vi "torres hanoi.vi"() -> ()   [LabVIEW 2020]
uses:
  <vilib>/Utility/miscctls.llb/LVPoint32TypeDef.ctl
  <vilib>/Utility/miscctls.llb/LVPositionTypeDef.ctl
  <vilib>/Utility/miscctls.llb/LVBoundsTypeDef.ctl
panel:
  out "?":string
  out "solucion de inicio a final 5":string
  out "solucion de inicio a final 4":string
  in  "?":bool
  out "solucion de inicio a final 3":string
  out "result":bool
  out "Position 1":T1
  out "# de movimientos":dbl
  out "Position 2":T1
  out "Position 3":T1
  out "Position 4":T1
  out "Position 5":T1
  out "Position":T1
  in  "seleccione  # de discos:":u16(ring) items=["3"=3, "4"=4, "5"=5]
  out "Coords":T2
  in  "?":bool
  out "disco5":bool
  out "disco4":bool
  out "disco3":bool
  out "disco2":bool
  out "disco1":bool
  out "final":bool
  out "medio":bool
  out "inicio":bool
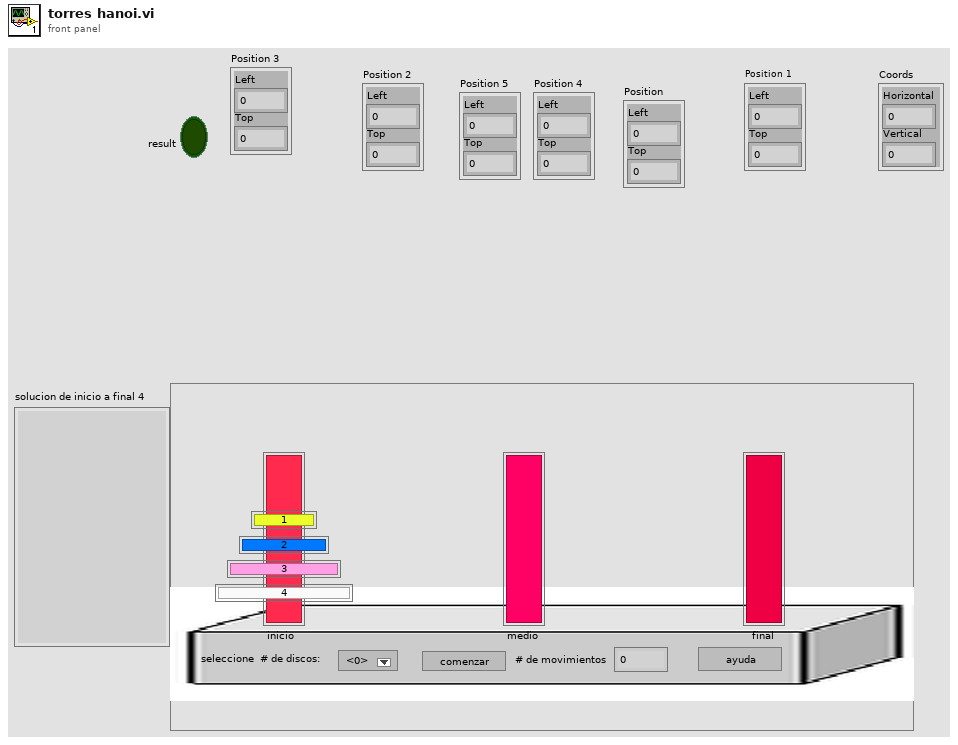
[diagram p1: front panel]
types:
  T1 = typedef "LVPositionTypeDef.ctl" = cluster{"Left":i32, "Top":i32}
  T2 = typedef "LVPoint32TypeDef.ctl" = cluster{"Horizontal":i32, "Vertical":i32}
  T3 = typedef "LVBoundsTypeDef.ctl" = cluster{"Width":u32, "Height":u32}
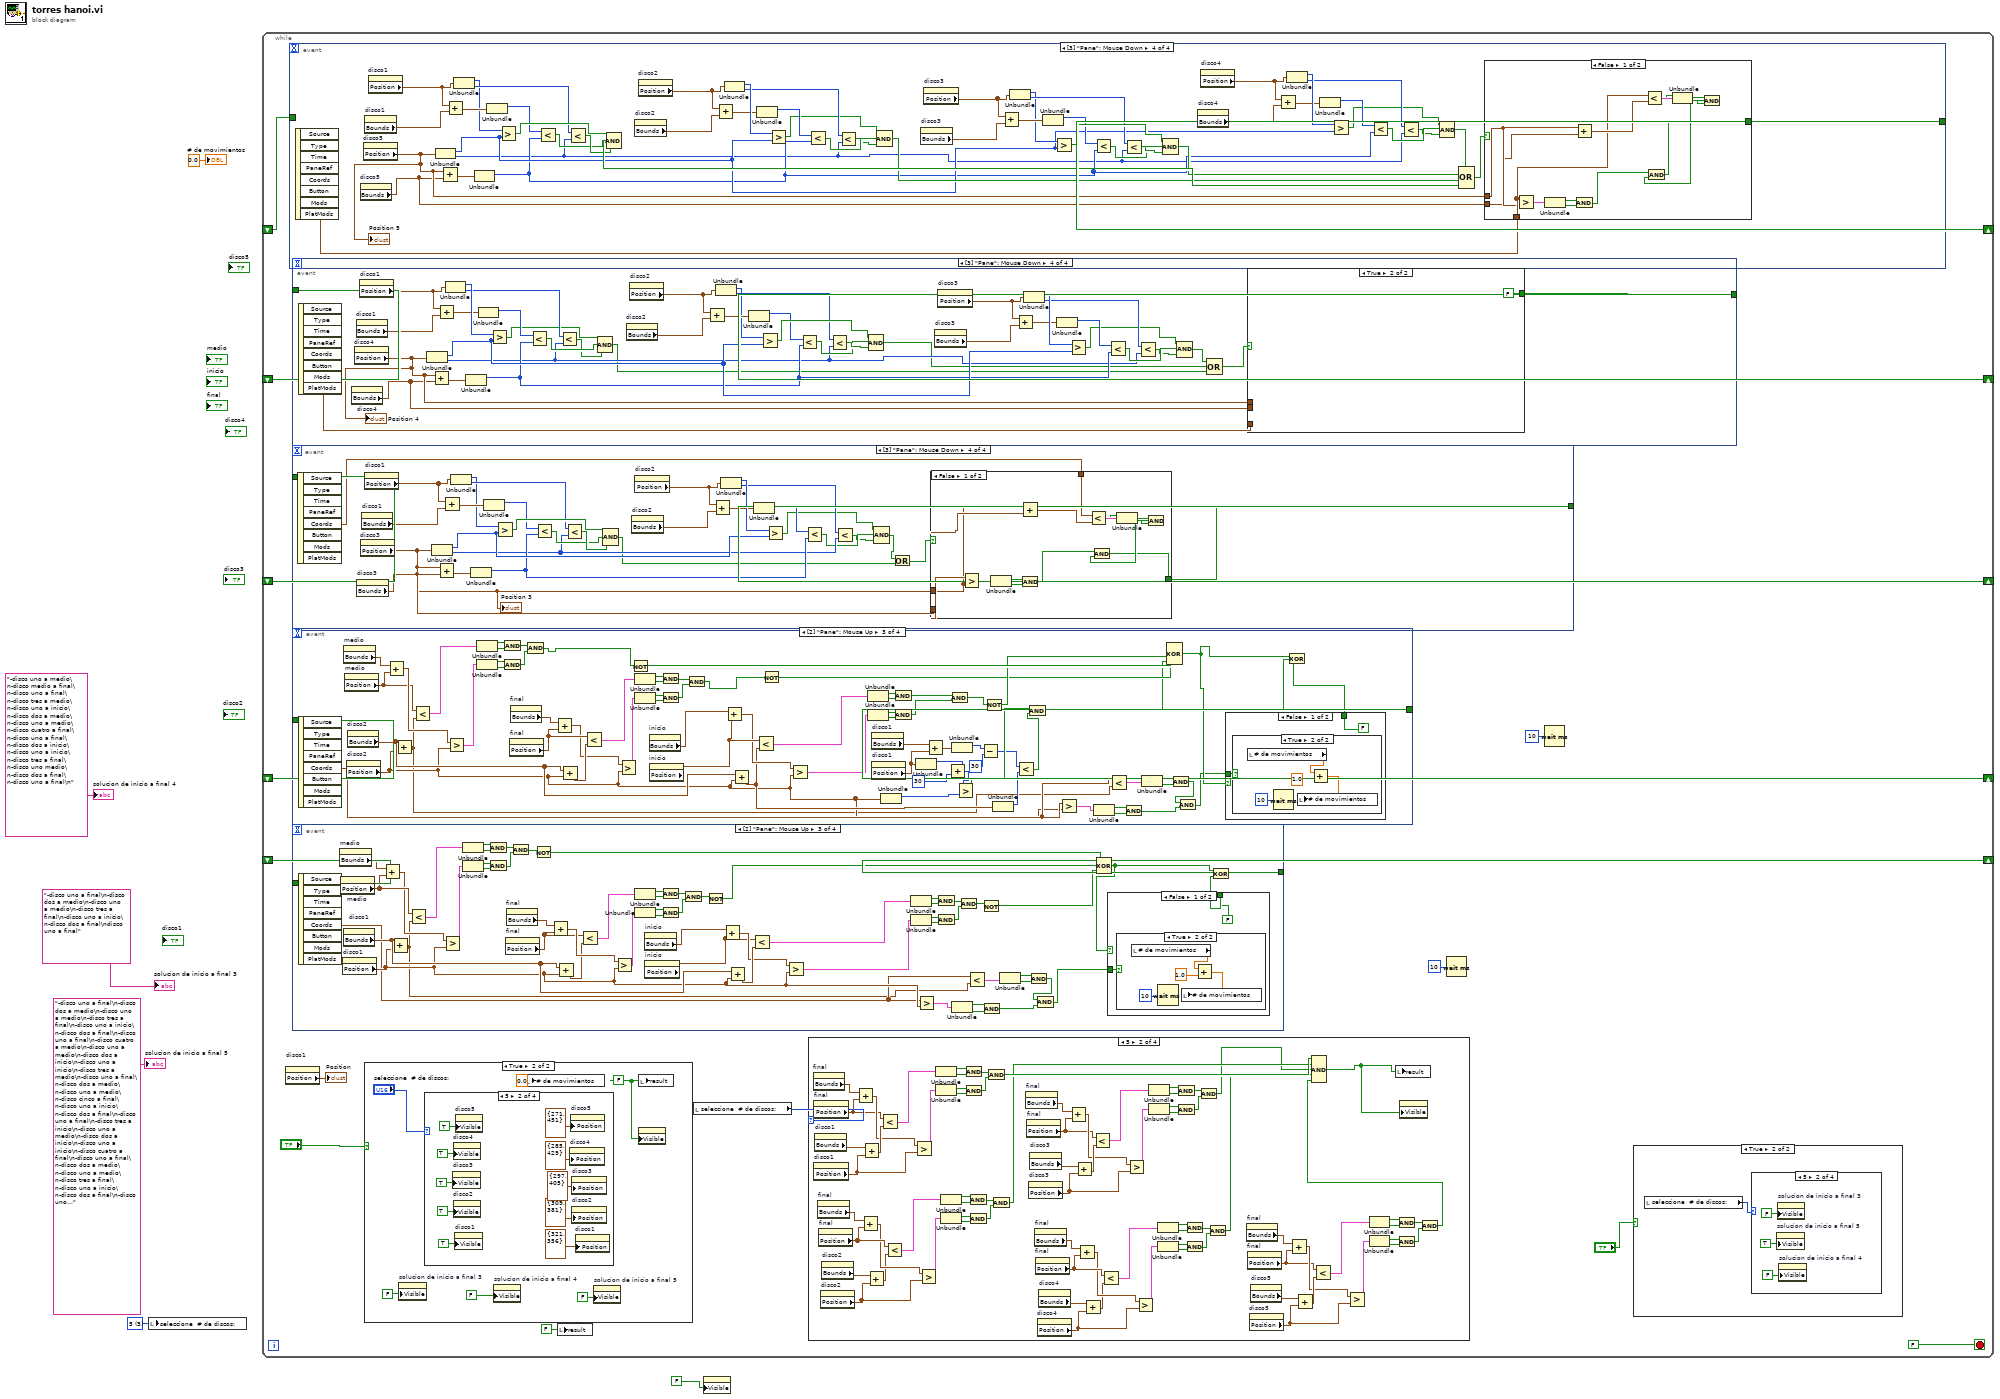
[diagram p0: block diagram]
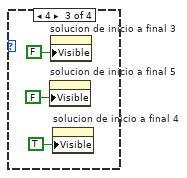
[diagram p4: hidden frame]
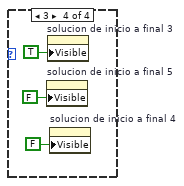
[diagram p5: hidden frame]
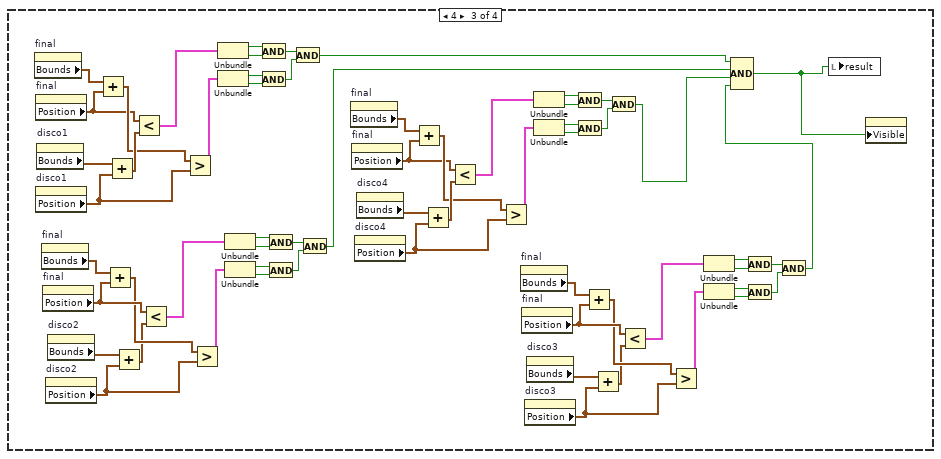
[diagram p7: hidden frame]
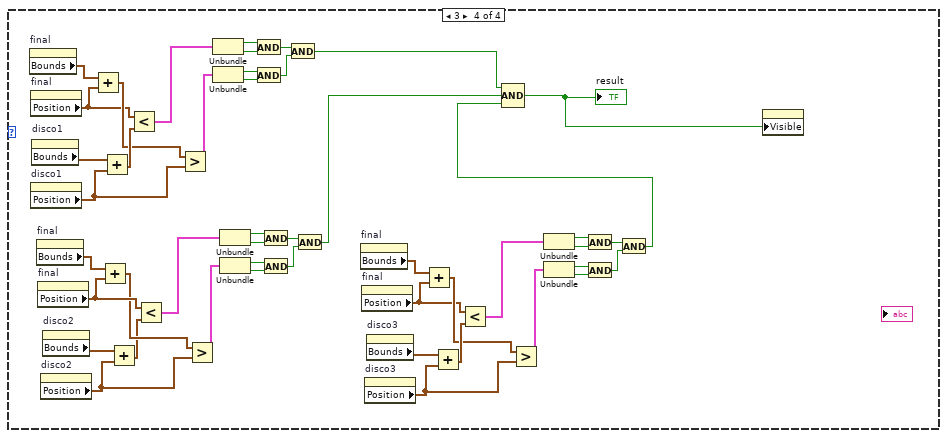
[diagram p8: hidden frame]
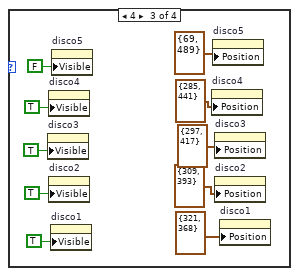
[diagram p11: hidden frame]
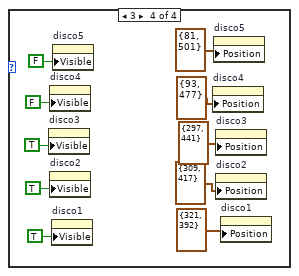
[diagram p12: hidden frame]
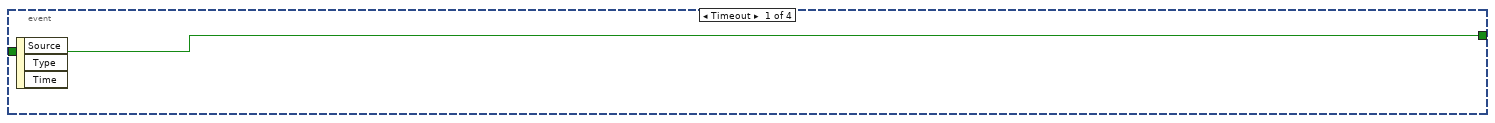
[diagram p13: hidden frame]
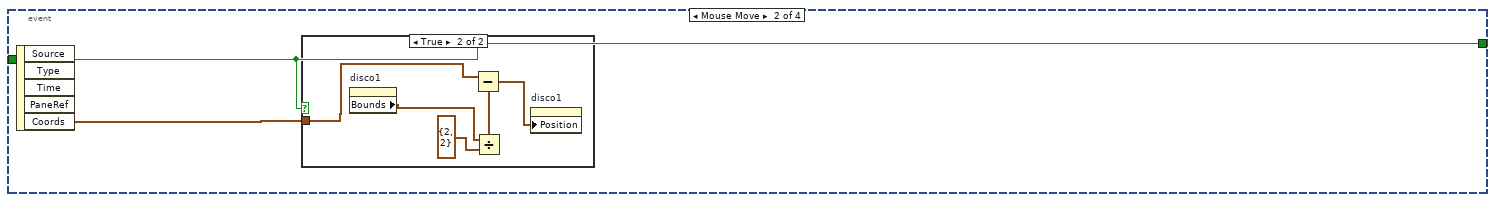
[diagram p14: hidden frame]
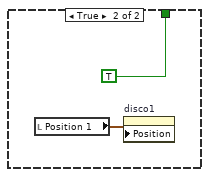
[diagram p17: hidden frame]
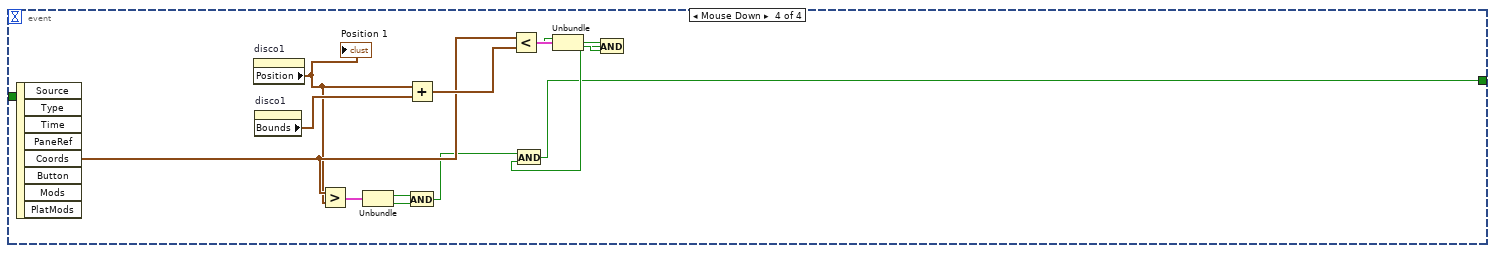
[diagram p18: hidden frame]
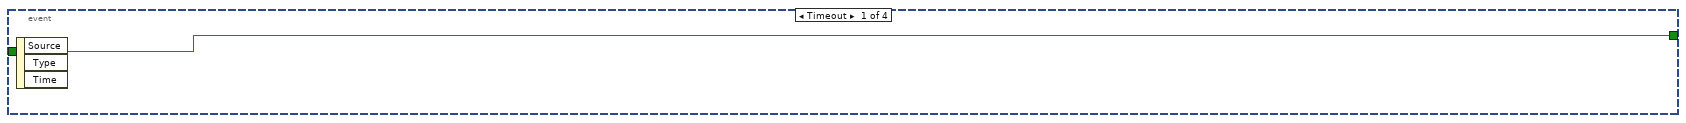
[diagram p19: hidden frame]
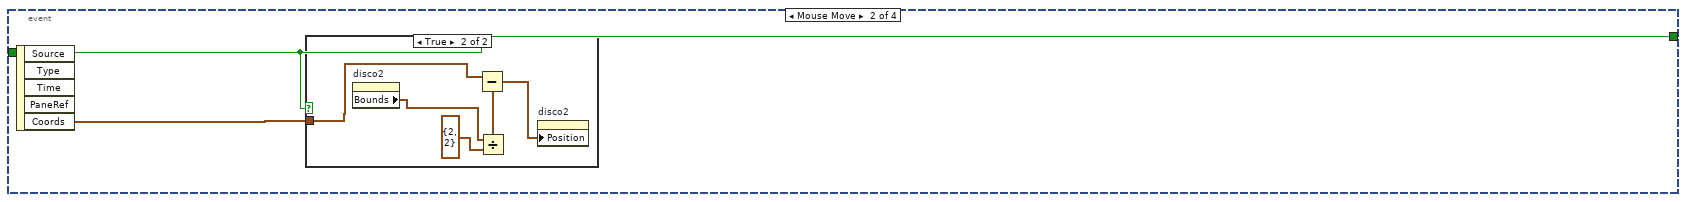
[diagram p20: hidden frame]
diagram:
  w4 = u16 5 items=["3"=3, "4"=4, "5"=5] ("seleccione  # de discos:")
  n1 = local write "seleccione  # de discos:"(w4) -> ()
  n2 = while {
    shift-right: [w22] -> _
    shift-left: _ -> [w23]
    shift-right: [w20] -> _
    shift-left: _ -> [w21]
    shift-right: [w18] -> _
    shift-left: _ -> [w19]
    shift-right: [w16] -> _
    shift-left: _ -> [w17]
    shift-right: [w14] -> _
    shift-left: _ -> [w15]
    stop <- FALSE stop-if-true
    n3 = property on="disco1" class="Bool (strict)"() -> ("Position"=→"Position":T1)  [unwired: 2 in, 2 out]
    n4 = event shown="[3] \"Pane\": Mouse Down" {
      selector: _ -> [_ _ _ _]
      dyn-events: _ -> [_ _ _ _]
      timeout: _ -> [_ _ _ _]
      tunnel: w23 -> [w768 w769 _ _]
      tunnel: [w768 w769 w840 w939] -> w22
      event Timeout {
        n5 = event-data() -> ()  [unwired: 1 in, 3 out]
      }
      event Mouse Move {
        n6 = event-data() -> ("Coords"=w770:T2)  [unwired: 1 in, 4 out]
        n7 = case shown="False" w769 {
          tunnel: w770 -> [_ w773]
          frame False {
          }
          frame True {
            n8 = property on="disco5" class="Bool (strict)"() -> ("Bounds"=w775:T3)  [unwired: 2 in, 2 out]
            n9 = Divide(x=w775, y=T3 {"Width"=2, "Height"=2}) -> (x/y=w772:cluster{"Width":dbl, "Height":dbl})
            n10 = Subtract(x=w773, y=w772) -> (x-y=w771:cluster{dbl, dbl})
            n11 = property on="disco5" class="Bool (strict)"("Position"=w771) -> ()  [unwired: 2 in, 2 out]
            "Coords" <- w773
          }
        }
      }
      event Mouse Up {
        n12 = event-data() -> ("Coords"=w778:T2)  [unwired: 1 in, 7 out]
        n13 = property on="medio" class="Bool (strict)"() -> ("Bounds"=w875:T3)  [unwired: 2 in, 2 out]
        n14 = property on="medio" class="Bool (strict)"() -> ("Position"=w874:T1)  [unwired: 2 in, 2 out]
        n15 = property on="disco5" class="Bool (strict)"() -> ("Position"=w777:T1)  [unwired: 2 in, 2 out]
        n16 = property on="disco5" class="Bool (strict)"() -> ("Bounds"=w846:T3)  [unwired: 2 in, 2 out]
        n17 = Add(x=w875, y=w874) -> (x+y=w873:T3)
        n18 = Add(x=w846, y=w777) -> (x+y=w776:T3)
        n19 = Less?(x=w874, y=w776) -> (x < y?=w877:cluster{bool, bool})
        n20 = Greater?(x=w873, y=w777) -> (0:w876:cluster{bool, bool})
        n21 = Unbundle(w877) -> (w881:bool, w880:bool)
        n22 = Unbundle(w876) -> (w883:bool, w882:bool)
        n23 = And(x=w881, y=w880) -> (x .and. y?=w878:bool)
        n24 = And(x=w883, y=w882) -> (x .and. y?=w879:bool)
        n25 = property on="final" class="Bool (strict)"() -> ("Position"=w859:T1)  [unwired: 2 in, 2 out]
        n26 = property on="final" class="Bool (strict)"() -> ("Bounds"=w860:T3)  [unwired: 2 in, 2 out]
        n27 = And(x=w878, y=w879) -> (x .and. y?=w872:bool)
        n28 = Not(x=w872) -> (.not. x?=w843:bool)
        n29 = Add(x=w860, y=w859) -> (x+y=w870:T3)
        n30 = Add(x=w846, y=w777) -> (x+y=w867:T3)
        n31 = Less?(x=w859, y=w867) -> (x < y?=w868:cluster{bool, bool})
        n32 = Greater?(x=w870, y=w777) -> (0:w869:cluster{bool, bool})
        n33 = Unbundle(w868) -> (w863:bool, w864:bool)
        n34 = Unbundle(w869) -> (w861:bool, w862:bool)
        n35 = property on="inicio" class="Bool (strict)"() -> ("Bounds"=w848:T3)  [unwired: 2 in, 2 out]
        n36 = property on="inicio" class="Bool (strict)"() -> ("Position"=w847:T1)  [unwired: 2 in, 2 out]
        n37 = And(x=w863, y=w864) -> (x .and. y?=w866:bool)
        n38 = And(x=w861, y=w862) -> (x .and. y?=w865:bool)
        n39 = And(x=w866, y=w865) -> (x .and. y?=w871:bool)
        n40 = Not(x=w871) -> (.not. x?=w844:bool)
        n41 = Add(x=w848, y=w847) -> (x+y=w850:T3)
        n42 = Add(x=w846, y=w777) -> (x+y=w828:T3)
        n43 = Less?(x=w847, y=w828) -> (x < y?=w852:cluster{bool, bool})
        n44 = Greater?(x=w850, y=w777) -> (0:w851:cluster{bool, bool})
        n45 = Unbundle(w852) -> (w856:bool, w855:bool)
        n46 = Unbundle(w851) -> (w858:bool, w857:bool)
        n47 = property on="disco1" class="Bool (strict)"() -> ("Bounds"=w834:T3)  [unwired: 2 in, 2 out]
        n48 = property on="disco1" class="Bool (strict)"() -> ("Position"=w835:T1)  [unwired: 2 in, 2 out]
        n49 = Unbundle(w777) -> ("Left"=w818:i32)  [unwired: 1 out]
        n50 = And(x=w856, y=w855) -> (x .and. y?=w853:bool)
        n51 = And(x=w858, y=w857) -> (x .and. y?=w854:bool)
        n52 = And(x=w853, y=w854) -> (x .and. y?=w849:bool)
        n53 = Unbundle(w835) -> ("Left"=w816:i32)  [unwired: 1 out]
        n54 = Add(x=w834, y=w835) -> (x+y=w836:T3)
        n55 = Not(x=w849) -> (.not. x?=w845:bool)
        n56 = Add(x=w816, y=30) -> (x+y=w814:i32)
        n57 = Greater?(x=w814, y=w818) -> (0:w830:bool)
        n58 = Unbundle(w836) -> ("Width"=w813:u32)  [unwired: 1 out]
        n59 = Subtract(x=w813, y=u32 30) -> (x-y=w811:u32)
        n60 = Unbundle(w828) -> ("Width"=w817:u32)  [unwired: 1 out]
        n61 = Less?(x=w811, y=w817) -> (x < y?=w829:bool)
        n62 = And(x=w830, y=w829) -> (x .and. y?=w788:bool)
        n63 = property on="disco2" class="Bool (strict)"() -> ("Bounds"=w833:T3)  [unwired: 2 in, 2 out]
        n64 = property on="disco2" class="Bool (strict)"() -> ("Position"=w832:T1)  [unwired: 2 in, 2 out]
        n65 = Unbundle(w832) -> ("Left"=w809:i32)  [unwired: 1 out]
        n66 = Add(x=w833, y=w832) -> (x+y=w831:T3)
        n67 = Add(x=w809, y=30) -> (x+y=w810:i32)
        n68 = Unbundle(w831) -> ("Width"=w807:u32)  [unwired: 1 out]
        n69 = Greater?(x=w810, y=w818) -> (0:w827:bool)
        n70 = Subtract(x=w807, y=u32 30) -> (x-y=w806:u32)
        n71 = Less?(x=w806, y=w817) -> (x < y?=w826:bool)
        n72 = And(x=w827, y=w826) -> (x .and. y?=w789:bool)
        n73 = property on="disco3" class="Bool (strict)"() -> ("Bounds"=w837:T3)  [unwired: 2 in, 2 out]
        n74 = property on="disco3" class="Bool (strict)"() -> ("Position"=w838:T1)  [unwired: 2 in, 2 out]
        n75 = Unbundle(w838) -> ("Left"=w804:i32)  [unwired: 1 out]
        n76 = Add(x=w837, y=w838) -> (x+y=w839:T3)
        n77 = Add(x=w804, y=30) -> (x+y=w803:i32)
        n78 = Unbundle(w839) -> ("Width"=w801:u32)  [unwired: 1 out]
        n79 = Greater?(x=w803, y=w818) -> (0:w825:bool)
        n80 = Subtract(x=w801, y=u32 30) -> (x-y=w800:u32)
        n81 = Less?(x=w800, y=w817) -> (x < y?=w824:bool)
        n82 = And(x=w825, y=w824) -> (x .and. y?=w790:bool)
        n83 = property on="disco4" class="Bool (strict)"() -> ("Bounds"=w821:T3)  [unwired: 2 in, 2 out]
        n84 = property on="disco4" class="Bool (strict)"() -> ("Position"=w820:T1)  [unwired: 2 in, 2 out]
        n85 = Unbundle(w820) -> ("Left"=w798:i32)  [unwired: 1 out]
        n86 = Add(x=w821, y=w820) -> (x+y=w819:T3)
        n87 = Add(x=w798, y=30) -> (x+y=w797:i32)
        n88 = Greater?(x=w797, y=w818) -> (0:w822:bool)
        n89 = Unbundle(w819) -> ("Width"=w795:u32)  [unwired: 1 out]
        n90 = Subtract(x=w795, y=u32 30) -> (x-y=w793:u32)
        n91 = Less?(x=w793, y=w817) -> (x < y?=w823:bool)
        n92 = And(x=w822, y=w823) -> (x .and. y?=w791:bool)
        n93 = Compound Arithmetic op=OR(w788, w789, w790, w791) -> (w792:bool)
        n94 = Greater?(x=w778, y=w777) -> (0:w787:cluster{bool, bool})
        n95 = Unbundle(w787) -> (w785:bool, w784:bool)
        n96 = Less?(x=w778, y=w776) -> (x < y?=w786:cluster{bool, bool})
        n97 = And(x=w785, y=w784) -> (x .and. y?=w780:bool)
        n98 = Unbundle(w786) -> (w783:bool, w782:bool)
        n99 = And(x=w783, y=w782) -> (x .and. y?=w781:bool)
        n100 = And(x=w781, y=w780) -> (x .and. y?=w779:bool)
        n101 = Compound Arithmetic op=XOR(w843, w844, w845, w792) -> (w841:bool)
        n102 = case shown="False" w841 {
          tunnel: [FALSE ("Accepted?") TRUE ("Accepted?")] -> w842
          tunnel: w779 -> [w884 _]
          frame False {
            n103 = case shown="True" w884 {
              frame False {
              }
              frame True {
                n104 = local read "# de movimientos"() -> (w888:dbl)
                n105 = Wait (ms)(milliseconds to wait=u32 10) -> ()  [unwired: 1 out]
                n106 = Add(x=w888, y=1.0) -> (x+y=w889:dbl)
                n107 = local write "# de movimientos"(w889) -> ()
              }
            }
          }
          frame True {
            n108 = local read "Position 5"() -> (w891:T1)
            n109 = property on="disco5" class="Bool (strict)"("Position"=w891) -> ()  [unwired: 2 in, 2 out]
          }
        }
        n110 = Exclusive Or(1:w842, 2:w841) -> (0:w840:bool)
      }
      event Mouse Down {
        n111 = event-data() -> ("Coords"=w940:T2)  [unwired: 1 in, 7 out]
        n112 = property on="disco5" class="Bool (strict)"() -> ("Bounds"=w906:T3)  [unwired: 2 in, 2 out]
        n113 = property on="disco5" class="Bool (strict)"() -> ("Position"=w907:T1)  [unwired: 2 in, 2 out]
        "Position 5" <- w907
        n114 = property on="disco1" class="Bool (strict)"() -> ("Bounds"=w917:T3)  [unwired: 2 in, 2 out]
        n115 = property on="disco1" class="Bool (strict)"() -> ("Position"=w918:T1)  [unwired: 2 in, 2 out]
        n116 = Unbundle(w907) -> ("Left"=w895:i32, "Top"=w893:i32)
        n117 = Add(x=w907, y=w906) -> (x+y=w921:T3)
        n118 = Add(x=w918, y=w917) -> (x+y=w920:T3)
        n119 = Unbundle(w918) -> ("Left"=w919:i32, "Top"=w923:i32)
        n120 = Unbundle(w921) -> ("Width"=w894:u32)  [unwired: 1 out]
        n121 = Unbundle(w920) -> ("Width"=w922:u32)  [unwired: 1 out]
        n122 = Greater?(x=w919, y=w895) -> (0:w924:bool)
        n123 = Less?(x=w922, y=w894) -> (x < y?=w925:bool)
        n124 = Less?(x=w923, y=w893) -> (x < y?=w926:bool)
        n125 = Compound Arithmetic op=AND(w924, w925, w926) -> (w938:bool)
        n126 = property on="disco2" class="Bool (strict)"() -> ("Bounds"=w916:T3)  [unwired: 2 in, 2 out]
        n127 = property on="disco2" class="Bool (strict)"() -> ("Position"=w915:T1)  [unwired: 2 in, 2 out]
        n128 = Add(x=w915, y=w916) -> (x+y=w913:T3)
        n129 = Unbundle(w915) -> ("Left"=w914:i32, "Top"=w911:i32)
        n130 = Unbundle(w913) -> ("Width"=w912:u32)  [unwired: 1 out]
        n131 = Greater?(x=w914, y=w895) -> (0:w910:bool)
        n132 = Less?(x=w912, y=w894) -> (x < y?=w909:bool)
        n133 = Less?(x=w911, y=w893) -> (x < y?=w908:bool)
        n134 = Compound Arithmetic op=AND(w910, w909, w908) -> (w937:bool)
        n135 = property on="disco3" class="Bool (strict)"() -> ("Bounds"=w927:T3)  [unwired: 2 in, 2 out]
        n136 = property on="disco3" class="Bool (strict)"() -> ("Position"=w928:T1)  [unwired: 2 in, 2 out]
        n137 = Add(x=w928, y=w927) -> (x+y=w930:T3)
        n138 = Unbundle(w928) -> ("Left"=w929:i32, "Top"=w932:i32)
        n139 = Unbundle(w930) -> ("Width"=w931:u32)  [unwired: 1 out]
        n140 = Greater?(x=w929, y=w895) -> (0:w933:bool)
        n141 = Less?(x=w931, y=w894) -> (x < y?=w934:bool)
        n142 = Less?(x=w932, y=w893) -> (x < y?=w935:bool)
        n143 = Compound Arithmetic op=AND(w933, w934, w935) -> (w936:bool)
        n144 = property on="disco4" class="Bool (strict)"() -> ("Bounds"=w905:T3)  [unwired: 2 in, 2 out]
        n145 = property on="disco4" class="Bool (strict)"() -> ("Position"=w904:T1)  [unwired: 2 in, 2 out]
        n146 = Add(x=w904, y=w905) -> (x+y=w902:T3)
        n147 = Unbundle(w904) -> ("Left"=w903:i32, "Top"=w900:i32)
        n148 = Unbundle(w902) -> ("Width"=w901:u32)  [unwired: 1 out]
        n149 = Greater?(x=w903, y=w895) -> (0:w899:bool)
        n150 = Less?(x=w901, y=w894) -> (x < y?=w898:bool)
        n151 = Less?(x=w900, y=w893) -> (x < y?=w897:bool)
        n152 = Compound Arithmetic op=AND(w899, w898, w897) -> (w896:bool)
        n153 = Compound Arithmetic op=OR(w896, w936, w937, w938) -> (w892:bool)
        n154 = case shown="False" w892 {
          tunnel: w940 -> [w952 _]
          tunnel: [w943 FALSE] -> w939
          tunnel: w907 -> [w942 _]
          tunnel: w906 -> [w941 _]
          frame False {
            n155 = Greater?(x=w952, y=w942) -> (0:w951:cluster{bool, bool})
            n156 = Unbundle(w951) -> (w947:bool, w946:bool)
            n157 = Add(x=w942, y=w941) -> (x+y=w953:T3)
            n158 = And(x=w947, y=w946) -> (x .and. y?=w944:bool)
            n159 = Less?(x=w952, y=w953) -> (x < y?=w950:cluster{bool, bool})
            n160 = Unbundle(w950) -> (w949:bool, w948:bool)
            n161 = And(x=w949, y=w948) -> (x .and. y?=w945:bool)
            n162 = And(x=w944, y=w945) -> (x .and. y?=w943:bool)
          }
          frame True {
          }
        }
      }
    }
    n163 = event shown="[3] \"Pane\": Mouse Down" {
      selector: _ -> [_ _ _ _]
      dyn-events: _ -> [_ _ _ _]
      timeout: _ -> [_ _ _ _]
      tunnel: w19 -> [w460 w461 _ _]
      tunnel: [w460 w461 w508 w587] -> w18
      event Timeout {
        n164 = event-data() -> ()  [unwired: 1 in, 3 out]
      }
      event Mouse Move {
        n165 = event-data() -> ("Coords"=w462:T2)  [unwired: 1 in, 4 out]
        n166 = case shown="False" w461 {
          tunnel: w462 -> [_ w466]
          frame False {
          }
          frame True {
            n167 = property on="disco3" class="Bool (strict)"() -> ("Bounds"=w464:T3)  [unwired: 2 in, 2 out]
            n168 = Divide(x=w464, y=T3 {"Width"=2, "Height"=2}) -> (x/y=w465:cluster{"Width":dbl, "Height":dbl})
            n169 = Subtract(x=w466, y=w465) -> (x-y=w463:cluster{dbl, dbl})
            n170 = property on="disco3" class="Bool (strict)"("Position"=w463) -> ()  [unwired: 2 in, 2 out]
          }
        }
      }
      event Mouse Up {
        n171 = event-data() -> ("Coords"=w470:T2)  [unwired: 1 in, 7 out]
        n172 = property on="medio" class="Bool (strict)"() -> ("Bounds"=w543:T3)  [unwired: 2 in, 2 out]
        n173 = property on="medio" class="Bool (strict)"() -> ("Position"=w542:T1)  [unwired: 2 in, 2 out]
        n174 = property on="disco3" class="Bool (strict)"() -> ("Position"=w469:T1)  [unwired: 2 in, 2 out]
        n175 = property on="disco3" class="Bool (strict)"() -> ("Bounds"=w514:T3)  [unwired: 2 in, 2 out]
        n176 = Add(x=w543, y=w542) -> (x+y=w541:T3)
        n177 = Add(x=w514, y=w469) -> (x+y=w468:T3)
        n178 = Less?(x=w542, y=w468) -> (x < y?=w545:cluster{bool, bool})
        n179 = Greater?(x=w541, y=w469) -> (0:w544:cluster{bool, bool})
        n180 = Unbundle(w545) -> (w549:bool, w548:bool)
        n181 = Unbundle(w544) -> (w551:bool, w550:bool)
        n182 = And(x=w549, y=w548) -> (x .and. y?=w546:bool)
        n183 = And(x=w551, y=w550) -> (x .and. y?=w547:bool)
        n184 = property on="final" class="Bool (strict)"() -> ("Position"=w527:T1)  [unwired: 2 in, 2 out]
        n185 = property on="final" class="Bool (strict)"() -> ("Bounds"=w528:T3)  [unwired: 2 in, 2 out]
        n186 = And(x=w546, y=w547) -> (x .and. y?=w540:bool)
        n187 = Not(x=w540) -> (.not. x?=w511:bool)
        n188 = Add(x=w528, y=w527) -> (x+y=w538:T3)
        n189 = Add(x=w514, y=w469) -> (x+y=w535:T3)
        n190 = Less?(x=w527, y=w535) -> (x < y?=w536:cluster{bool, bool})
        n191 = Greater?(x=w538, y=w469) -> (0:w537:cluster{bool, bool})
        n192 = Unbundle(w536) -> (w531:bool, w532:bool)
        n193 = Unbundle(w537) -> (w529:bool, w530:bool)
        n194 = property on="inicio" class="Bool (strict)"() -> ("Bounds"=w516:T3)  [unwired: 2 in, 2 out]
        n195 = property on="inicio" class="Bool (strict)"() -> ("Position"=w515:T1)  [unwired: 2 in, 2 out]
        n196 = And(x=w531, y=w532) -> (x .and. y?=w534:bool)
        n197 = And(x=w529, y=w530) -> (x .and. y?=w533:bool)
        n198 = And(x=w534, y=w533) -> (x .and. y?=w539:bool)
        n199 = Not(x=w539) -> (.not. x?=w512:bool)
        n200 = Add(x=w516, y=w515) -> (x+y=w518:T3)
        n201 = Add(x=w514, y=w469) -> (x+y=w504:T3)
        n202 = Less?(x=w515, y=w504) -> (x < y?=w520:cluster{bool, bool})
        n203 = Greater?(x=w518, y=w469) -> (0:w519:cluster{bool, bool})
        n204 = Unbundle(w520) -> (w524:bool, w523:bool)
        n205 = Unbundle(w519) -> (w526:bool, w525:bool)
        n206 = And(x=w524, y=w523) -> (x .and. y?=w521:bool)
        n207 = And(x=w526, y=w525) -> (x .and. y?=w522:bool)
        n208 = And(x=w521, y=w522) -> (x .and. y?=w517:bool)
        n209 = property on="disco1" class="Bool (strict)"() -> ("Bounds"=w505:T3)  [unwired: 2 in, 2 out]
        n210 = property on="disco1" class="Bool (strict)"() -> ("Position"=w506:T1)  [unwired: 2 in, 2 out]
        n211 = Unbundle(w469) -> ("Left"=w498:i32)  [unwired: 1 out]
        n212 = Not(x=w517) -> (.not. x?=w513:bool)
        n213 = Unbundle(w506) -> ("Left"=w494:i32)  [unwired: 1 out]
        n214 = Add(x=w505, y=w506) -> (x+y=w507:T3)
        n215 = Add(x=w494, y=30) -> (x+y=w493:i32)
        n216 = Unbundle(w507) -> ("Width"=w490:u32)  [unwired: 1 out]
        n217 = Greater?(x=w493, y=w498) -> (0:w503:bool)
        n218 = Subtract(x=w490, y=u32 30) -> (x-y=w491:u32)
        n219 = Unbundle(w504) -> ("Width"=w497:u32)  [unwired: 1 out]
        n220 = Less?(x=w491, y=w497) -> (x < y?=w502:bool)
        n221 = And(x=w503, y=w502) -> (x .and. y?=w481:bool)
        n222 = property on="disco2" class="Bool (strict)"() -> ("Bounds"=w501:T3)  [unwired: 2 in, 2 out]
        n223 = property on="disco2" class="Bool (strict)"() -> ("Position"=w500:T1)  [unwired: 2 in, 2 out]
        n224 = Unbundle(w500) -> ("Left"=w488:i32)  [unwired: 1 out]
        n225 = Add(x=w501, y=w500) -> (x+y=w499:T3)
        n226 = Add(x=w488, y=30) -> (x+y=w487:i32)
        n227 = Unbundle(w499) -> ("Width"=w485:u32)  [unwired: 1 out]
        n228 = Greater?(x=w487, y=w498) -> (0:w495:bool)
        n229 = Subtract(x=w485, y=u32 30) -> (x-y=w484:u32)
        n230 = Less?(x=w484, y=w497) -> (x < y?=w496:bool)
        n231 = And(x=w495, y=w496) -> (x .and. y?=w482:bool)
        n232 = Or(x=w481, y=w482) -> (x .or. y?=w480:bool)
        n233 = Greater?(x=w470, y=w469) -> (0:w479:cluster{bool, bool})
        n234 = Unbundle(w479) -> (w477:bool, w476:bool)
        n235 = Less?(x=w470, y=w468) -> (x < y?=w478:cluster{bool, bool})
        n236 = And(x=w477, y=w476) -> (x .and. y?=w472:bool)
        n237 = Unbundle(w478) -> (w475:bool, w474:bool)
        n238 = And(x=w475, y=w474) -> (x .and. y?=w473:bool)
        n239 = And(x=w473, y=w472) -> (x .and. y?=w471:bool)
        n240 = Compound Arithmetic op=XOR(w511, w512, w513, w480) -> (w509:bool)
        n241 = case shown="False" w509 {
          tunnel: [FALSE ("Accepted?") TRUE ("Accepted?")] -> w510
          tunnel: w471 -> [w552 _]
          frame False {
            n242 = case shown="True" w552 {
              frame False {
              }
              frame True {
                n243 = local read "# de movimientos"() -> (w556:dbl)
                n244 = Wait (ms)(milliseconds to wait=u32 10) -> ()  [unwired: 1 out]
                n245 = Add(x=w556, y=1.0) -> (x+y=w557:dbl)
                n246 = local write "# de movimientos"(w557) -> ()
              }
            }
          }
          frame True {
            n247 = local read "Position 3"() -> (w559:T1)
            n248 = property on="disco3" class="Bool (strict)"("Position"=w559) -> ()  [unwired: 2 in, 2 out]
          }
        }
        n249 = Exclusive Or(1:w510, 2:w509) -> (0:w508:bool)
      }
      event Mouse Down {
        n250 = event-data() -> ("Coords"=w588:T2)  [unwired: 1 in, 7 out]
        n251 = property on="disco3" class="Bool (strict)"() -> ("Bounds"=w576:T3)  [unwired: 2 in, 2 out]
        n252 = property on="disco3" class="Bool (strict)"() -> ("Position"=w575:T1)  [unwired: 2 in, 2 out]
        "Position 3" <- w575
        n253 = property on="disco1" class="Bool (strict)"() -> ("Bounds"=w577:T3)  [unwired: 2 in, 2 out]
        n254 = property on="disco1" class="Bool (strict)"() -> ("Position"=w578:T1)  [unwired: 2 in, 2 out]
        n255 = Unbundle(w575) -> ("Left"=w567:i32, "Top"=w565:i32)
        n256 = Add(x=w575, y=w576) -> (x+y=w581:T3)
        n257 = Add(x=w578, y=w577) -> (x+y=w580:T3)
        n258 = Unbundle(w578) -> ("Left"=w579:i32, "Top"=w583:i32)
        n259 = Unbundle(w581) -> ("Width"=w566:u32)  [unwired: 1 out]
        n260 = Unbundle(w580) -> ("Width"=w582:u32)  [unwired: 1 out]
        n261 = Greater?(x=w579, y=w567) -> (0:w584:bool)
        n262 = Less?(x=w582, y=w566) -> (x < y?=w585:bool)
        n263 = Less?(x=w583, y=w565) -> (x < y?=w586:bool)
        n264 = Compound Arithmetic op=AND(w584, w585, w586) -> (w560:bool)
        n265 = property on="disco2" class="Bool (strict)"() -> ("Bounds"=w574:T3)  [unwired: 2 in, 2 out]
        n266 = property on="disco2" class="Bool (strict)"() -> ("Position"=w573:T1)  [unwired: 2 in, 2 out]
        n267 = Add(x=w573, y=w574) -> (x+y=w571:T3)
        n268 = Unbundle(w573) -> ("Left"=w572:i32, "Top"=w569:i32)
        n269 = Unbundle(w571) -> ("Width"=w570:u32)  [unwired: 1 out]
        n270 = Greater?(x=w572, y=w567) -> (0:w568:bool)
        n271 = Less?(x=w570, y=w566) -> (x < y?=w564:bool)
        n272 = Less?(x=w569, y=w565) -> (x < y?=w563:bool)
        n273 = Compound Arithmetic op=AND(w568, w564, w563) -> (w561:bool)
        n274 = Or(x=w561, y=w560) -> (x .or. y?=w562:bool)
        n275 = case shown="False" w562 {
          tunnel: w588 -> [w592 _]
          tunnel: [w591 FALSE] -> w587
          tunnel: w576 -> [w590 _]
          tunnel: w575 -> [w589 _]
          frame False {
            n276 = Greater?(x=w592, y=w589) -> (0:w600:cluster{bool, bool})
            n277 = Unbundle(w600) -> (w596:bool, w595:bool)
            n278 = Add(x=w589, y=w590) -> (x+y=w601:T3)
            n279 = And(x=w596, y=w595) -> (x .and. y?=w593:bool)
            n280 = Less?(x=w592, y=w601) -> (x < y?=w599:cluster{bool, bool})
            n281 = Unbundle(w599) -> (w598:bool, w597:bool)
            n282 = And(x=w598, y=w597) -> (x .and. y?=w594:bool)
            n283 = And(x=w593, y=w594) -> (x .and. y?=w591:bool)
          }
          frame True {
          }
        }
      }
    }
    n284 = event shown="[3] \"Pane\": Mouse Down" {
      selector: _ -> [_ _ _ _]
      dyn-events: _ -> [_ _ _ _]
      timeout: _ -> [_ _ _ _]
      tunnel: w21 -> [w603 w604 _ _]
      tunnel: [w603 w604 w664 w752] -> w20
      event Timeout {
        n285 = event-data() -> ()  [unwired: 1 in, 3 out]
      }
      event Mouse Move {
        n286 = event-data() -> ("Coords"=w605:T2)  [unwired: 1 in, 4 out]
        n287 = case shown="False" w604 {
          tunnel: w605 -> [_ w606]
          frame False {
          }
          frame True {
            n288 = property on="disco4" class="Bool (strict)"() -> ("Bounds"=w608:T3)  [unwired: 2 in, 2 out]
            n289 = Divide(x=w608, y=T3 {"Width"=2, "Height"=2}) -> (x/y=w609:cluster{"Width":dbl, "Height":dbl})
            n290 = Subtract(x=w606, y=w609) -> (x-y=w607:cluster{dbl, dbl})
            n291 = property on="disco4" class="Bool (strict)"("Position"=w607) -> ()  [unwired: 2 in, 2 out]
          }
        }
      }
      event Mouse Up {
        n292 = event-data() -> ("Coords"=w613:T2)  [unwired: 1 in, 7 out]
        n293 = property on="medio" class="Bool (strict)"() -> ("Bounds"=w673:T3)  [unwired: 2 in, 2 out]
        n294 = property on="medio" class="Bool (strict)"() -> ("Position"=w674:T1)  [unwired: 2 in, 2 out]
        n295 = property on="disco4" class="Bool (strict)"() -> ("Position"=w612:T1)  [unwired: 2 in, 2 out]
        n296 = property on="disco4" class="Bool (strict)"() -> ("Bounds"=w702:T3)  [unwired: 2 in, 2 out]
        n297 = Add(x=w673, y=w674) -> (x+y=w675:T3)
        n298 = Add(x=w702, y=w612) -> (x+y=w611:T3)
        n299 = Less?(x=w674, y=w611) -> (x < y?=w671:cluster{bool, bool})
        n300 = Greater?(x=w675, y=w612) -> (0:w672:cluster{bool, bool})
        n301 = Unbundle(w671) -> (w667:bool, w668:bool)
        n302 = Unbundle(w672) -> (w665:bool, w666:bool)
        n303 = And(x=w667, y=w668) -> (x .and. y?=w670:bool)
        n304 = And(x=w665, y=w666) -> (x .and. y?=w669:bool)
        n305 = property on="final" class="Bool (strict)"() -> ("Position"=w689:T1)  [unwired: 2 in, 2 out]
        n306 = property on="final" class="Bool (strict)"() -> ("Bounds"=w688:T3)  [unwired: 2 in, 2 out]
        n307 = And(x=w670, y=w669) -> (x .and. y?=w676:bool)
        n308 = Not(x=w676) -> (.not. x?=w704:bool)
        n309 = Add(x=w688, y=w689) -> (x+y=w678:T3)
        n310 = Add(x=w702, y=w612) -> (x+y=w681:T3)
        n311 = Less?(x=w689, y=w681) -> (x < y?=w680:cluster{bool, bool})
        n312 = Greater?(x=w678, y=w612) -> (0:w679:cluster{bool, bool})
        n313 = Unbundle(w680) -> (w685:bool, w684:bool)
        n314 = Unbundle(w679) -> (w687:bool, w686:bool)
        n315 = property on="inicio" class="Bool (strict)"() -> ("Bounds"=w700:T3)  [unwired: 2 in, 2 out]
        n316 = property on="inicio" class="Bool (strict)"() -> ("Position"=w701:T1)  [unwired: 2 in, 2 out]
        n317 = And(x=w685, y=w684) -> (x .and. y?=w682:bool)
        n318 = And(x=w687, y=w686) -> (x .and. y?=w683:bool)
        n319 = And(x=w682, y=w683) -> (x .and. y?=w677:bool)
        n320 = Not(x=w677) -> (.not. x?=w703:bool)
        n321 = Add(x=w700, y=w701) -> (x+y=w698:T3)
        n322 = Add(x=w702, y=w612) -> (x+y=w653:T3)
        n323 = Less?(x=w701, y=w653) -> (x < y?=w696:cluster{bool, bool})
        n324 = Greater?(x=w698, y=w612) -> (0:w697:cluster{bool, bool})
        n325 = Unbundle(w696) -> (w692:bool, w693:bool)
        n326 = Unbundle(w697) -> (w690:bool, w691:bool)
        n327 = And(x=w692, y=w693) -> (x .and. y?=w695:bool)
        n328 = And(x=w690, y=w691) -> (x .and. y?=w694:bool)
        n329 = And(x=w695, y=w694) -> (x .and. y?=w699:bool)
        n330 = property on="disco1" class="Bool (strict)"() -> ("Bounds"=w660:T3)  [unwired: 2 in, 2 out]
        n331 = property on="disco1" class="Bool (strict)"() -> ("Position"=w659:T1)  [unwired: 2 in, 2 out]
        n332 = Unbundle(w612) -> ("Left"=w649:i32)  [unwired: 1 out]
        n333 = Not(x=w699) -> (.not. x?=w624:bool)
        n334 = Unbundle(w659) -> ("Left"=w645:i32)  [unwired: 1 out]
        n335 = Add(x=w660, y=w659) -> (x+y=w658:T3)
        n336 = Add(x=w645, y=30) -> (x+y=w643:i32)
        n337 = Unbundle(w658) -> ("Width"=w642:u32)  [unwired: 1 out]
        n338 = Greater?(x=w643, y=w649) -> (0:w655:bool)
        n339 = Subtract(x=w642, y=u32 30) -> (x-y=w641:u32)
        n340 = Unbundle(w653) -> ("Width"=w648:u32)  [unwired: 1 out]
        n341 = Less?(x=w641, y=w648) -> (x < y?=w654:bool)
        n342 = And(x=w655, y=w654) -> (x .and. y?=w625:bool)
        n343 = property on="disco2" class="Bool (strict)"() -> ("Bounds"=w661:T3)  [unwired: 2 in, 2 out]
        n344 = property on="disco2" class="Bool (strict)"() -> ("Position"=w662:T1)  [unwired: 2 in, 2 out]
        n345 = Unbundle(w662) -> ("Left"=w638:i32)  [unwired: 1 out]
        n346 = Add(x=w661, y=w662) -> (x+y=w663:T3)
        n347 = Add(x=w638, y=30) -> (x+y=w639:i32)
        n348 = Unbundle(w663) -> ("Width"=w636:u32)  [unwired: 1 out]
        n349 = Greater?(x=w639, y=w649) -> (0:w657:bool)
        n350 = Subtract(x=w636, y=u32 30) -> (x-y=w634:u32)
        n351 = Less?(x=w634, y=w648) -> (x < y?=w656:bool)
        n352 = And(x=w657, y=w656) -> (x .and. y?=w626:bool)
        n353 = property on="disco3" class="Bool (strict)"() -> ("Bounds"=w652:T3)  [unwired: 2 in, 2 out]
        n354 = property on="disco3" class="Bool (strict)"() -> ("Position"=w651:T1)  [unwired: 2 in, 2 out]
        n355 = Unbundle(w651) -> ("Left"=w633:i32)  [unwired: 1 out]
        n356 = Add(x=w652, y=w651) -> (x+y=w650:T3)
        n357 = Add(x=w633, y=30) -> (x+y=w632:i32)
        n358 = Unbundle(w650) -> ("Width"=w630:u32)  [unwired: 1 out]
        n359 = Greater?(x=w632, y=w649) -> (0:w647:bool)
        n360 = Subtract(x=w630, y=u32 30) -> (x-y=w629:u32)
        n361 = Less?(x=w629, y=w648) -> (x < y?=w646:bool)
        n362 = And(x=w647, y=w646) -> (x .and. y?=w627:bool)
        n363 = Compound Arithmetic op=OR(w625, w626, w627) -> (w623:bool)
        n364 = Greater?(x=w613, y=w612) -> (0:w615:cluster{bool, bool})
        n365 = Unbundle(w615) -> (w617:bool, w618:bool)
        n366 = Less?(x=w613, y=w611) -> (x < y?=w616:cluster{bool, bool})
        n367 = And(x=w617, y=w618) -> (x .and. y?=w622:bool)
        n368 = Unbundle(w616) -> (w619:bool, w620:bool)
        n369 = And(x=w619, y=w620) -> (x .and. y?=w621:bool)
        n370 = And(x=w621, y=w622) -> (x .and. y?=w614:bool)
        n371 = Compound Arithmetic op=XOR(w704, w703, w624, w623) -> (w706:bool)
        n372 = case shown="False" w706 {
          tunnel: [FALSE ("Accepted?") TRUE ("Accepted?")] -> w705
          tunnel: w614 -> [w707 _]
          frame False {
            n373 = case shown="True" w707 {
              frame False {
              }
              frame True {
                n374 = local read "# de movimientos"() -> (w711:dbl)
                n375 = Wait (ms)(milliseconds to wait=u32 10) -> ()  [unwired: 1 out]
                n376 = Add(x=w711, y=1.0) -> (x+y=w712:dbl)
                n377 = local write "# de movimientos"(w712) -> ()
              }
            }
          }
          frame True {
            n378 = local read "Position 4"() -> (w714:T1)
            n379 = property on="disco4" class="Bool (strict)"("Position"=w714) -> ()  [unwired: 2 in, 2 out]
          }
        }
        n380 = Exclusive Or(1:w705, 2:w706) -> (0:w664:bool)
      }
      event Mouse Down {
        n381 = event-data() -> ("Coords"=w753:T2)  [unwired: 1 in, 7 out]
        n382 = property on="disco4" class="Bool (strict)"() -> ("Bounds"=w731:T3)  [unwired: 2 in, 2 out]
        n383 = property on="disco4" class="Bool (strict)"() -> ("Position"=w732:T1)  [unwired: 2 in, 2 out]
        "Position 4" <- w732
        n384 = property on="disco1" class="Bool (strict)"() -> ("Bounds"=w742:T3)  [unwired: 2 in, 2 out]
        n385 = property on="disco1" class="Bool (strict)"() -> ("Position"=w741:T1)  [unwired: 2 in, 2 out]
        n386 = Unbundle(w732) -> ("Left"=w721:i32, "Top"=w719:i32)
        n387 = Add(x=w732, y=w731) -> (x+y=w738:T3)
        n388 = Add(x=w741, y=w742) -> (x+y=w739:T3)
        n389 = Unbundle(w741) -> ("Left"=w740:i32, "Top"=w736:i32)
        n390 = Unbundle(w738) -> ("Width"=w720:u32)  [unwired: 1 out]
        n391 = Unbundle(w739) -> ("Width"=w737:u32)  [unwired: 1 out]
        n392 = Greater?(x=w740, y=w721) -> (0:w735:bool)
        n393 = Less?(x=w737, y=w720) -> (x < y?=w734:bool)
        n394 = Less?(x=w736, y=w719) -> (x < y?=w733:bool)
        n395 = Compound Arithmetic op=AND(w735, w734, w733) -> (w715:bool)
        n396 = property on="disco2" class="Bool (strict)"() -> ("Bounds"=w743:T3)  [unwired: 2 in, 2 out]
        n397 = property on="disco2" class="Bool (strict)"() -> ("Position"=w744:T1)  [unwired: 2 in, 2 out]
        n398 = Add(x=w744, y=w743) -> (x+y=w746:T3)
        n399 = Unbundle(w744) -> ("Left"=w745:i32, "Top"=w748:i32)
        n400 = Unbundle(w746) -> ("Width"=w747:u32)  [unwired: 1 out]
        n401 = Greater?(x=w745, y=w721) -> (0:w749:bool)
        n402 = Less?(x=w747, y=w720) -> (x < y?=w750:bool)
        n403 = Less?(x=w748, y=w719) -> (x < y?=w751:bool)
        n404 = Compound Arithmetic op=AND(w749, w750, w751) -> (w716:bool)
        n405 = property on="disco3" class="Bool (strict)"() -> ("Bounds"=w730:T3)  [unwired: 2 in, 2 out]
        n406 = property on="disco3" class="Bool (strict)"() -> ("Position"=w729:T1)  [unwired: 2 in, 2 out]
        n407 = Add(x=w729, y=w730) -> (x+y=w727:T3)
        n408 = Unbundle(w729) -> ("Left"=w728:i32, "Top"=w725:i32)
        n409 = Unbundle(w727) -> ("Width"=w726:u32)  [unwired: 1 out]
        n410 = Greater?(x=w728, y=w721) -> (0:w724:bool)
        n411 = Less?(x=w726, y=w720) -> (x < y?=w723:bool)
        n412 = Less?(x=w725, y=w719) -> (x < y?=w722:bool)
        n413 = Compound Arithmetic op=AND(w724, w723, w722) -> (w717:bool)
        n414 = Compound Arithmetic op=OR(w717, w716, w715) -> (w718:bool)
        n415 = case shown="True" w718 {
          tunnel: w753 -> [w765 _]
          tunnel: [w756 FALSE] -> w752
          tunnel: w732 -> [w755 _]
          tunnel: w731 -> [w754 _]
          frame False {
            n416 = Greater?(x=w765, y=w755) -> (0:w764:cluster{bool, bool})
            n417 = Unbundle(w764) -> (w760:bool, w759:bool)
            n418 = Add(x=w755, y=w754) -> (x+y=w766:T3)
            n419 = And(x=w760, y=w759) -> (x .and. y?=w757:bool)
            n420 = Less?(x=w765, y=w766) -> (x < y?=w763:cluster{bool, bool})
            n421 = Unbundle(w763) -> (w762:bool, w761:bool)
            n422 = And(x=w762, y=w761) -> (x .and. y?=w758:bool)
            n423 = And(x=w757, y=w758) -> (x .and. y?=w756:bool)
          }
          frame True {
          }
        }
      }
    }
    n424 = event shown="[2] \"Pane\": Mouse Up" {
      selector: _ -> [_ _ _ _]
      dyn-events: _ -> [_ _ _ _]
      timeout: _ -> [_ _ _ _]
      tunnel: w17 -> [w340 w341 _ _]
      tunnel: [w340 w341 w379 w428] -> w16
      event Timeout {
        n425 = event-data() -> ()  [unwired: 1 in, 3 out]
      }
      event Mouse Move {
        n426 = event-data() -> ("Coords"=w342:T2)  [unwired: 1 in, 4 out]
        n427 = case shown="True" w341 {
          tunnel: w342 -> [_ w346]
          frame False {
          }
          frame True {
            n428 = property on="disco2" class="Bool (strict)"() -> ("Bounds"=w344:T3)  [unwired: 2 in, 2 out]
            n429 = Divide(x=w344, y=T3 {"Width"=2, "Height"=2}) -> (x/y=w345:cluster{"Width":dbl, "Height":dbl})
            n430 = Subtract(x=w346, y=w345) -> (x-y=w343:cluster{dbl, dbl})
            n431 = property on="disco2" class="Bool (strict)"("Position"=w343) -> ()  [unwired: 2 in, 2 out]
          }
        }
      }
      event Mouse Up {
        n432 = event-data() -> ("Coords"=w350:T2)  [unwired: 1 in, 7 out]
        n433 = property on="medio" class="Bool (strict)"() -> ("Bounds"=w388:T3)  [unwired: 2 in, 2 out]
        n434 = property on="medio" class="Bool (strict)"() -> ("Position"=w389:T1)  [unwired: 2 in, 2 out]
        n435 = property on="disco2" class="Bool (strict)"() -> ("Position"=w349:T1)  [unwired: 2 in, 2 out]
        n436 = property on="disco2" class="Bool (strict)"() -> ("Bounds"=w414:T3)  [unwired: 2 in, 2 out]
        n437 = Add(x=w388, y=w389) -> (x+y=w390:T3)
        n438 = Add(x=w414, y=w349) -> (x+y=w348:T3)
        n439 = Less?(x=w389, y=w348) -> (x < y?=w386:cluster{bool, bool})
        n440 = Greater?(x=w390, y=w349) -> (0:w387:cluster{bool, bool})
        n441 = Unbundle(w386) -> (w382:bool, w383:bool)
        n442 = Unbundle(w387) -> (w380:bool, w381:bool)
        n443 = And(x=w382, y=w383) -> (x .and. y?=w385:bool)
        n444 = And(x=w380, y=w381) -> (x .and. y?=w384:bool)
        n445 = property on="final" class="Bool (strict)"() -> ("Position"=w402:T1)  [unwired: 2 in, 2 out]
        n446 = property on="final" class="Bool (strict)"() -> ("Bounds"=w401:T3)  [unwired: 2 in, 2 out]
        n447 = And(x=w385, y=w384) -> (x .and. y?=w377:bool)
        n448 = Add(x=w401, y=w402) -> (x+y=w391:T3)
        n449 = Add(x=w414, y=w349) -> (x+y=w394:T3)
        n450 = Less?(x=w402, y=w394) -> (x < y?=w393:cluster{bool, bool})
        n451 = Greater?(x=w391, y=w349) -> (0:w392:cluster{bool, bool})
        n452 = Not(x=w377) -> (.not. x?=w416:bool)
        n453 = Unbundle(w393) -> (w398:bool, w397:bool)
        n454 = Unbundle(w392) -> (w400:bool, w399:bool)
        n455 = property on="inicio" class="Bool (strict)"() -> ("Bounds"=w412:T3)  [unwired: 2 in, 2 out]
        n456 = property on="inicio" class="Bool (strict)"() -> ("Position"=w413:T1)  [unwired: 2 in, 2 out]
        n457 = And(x=w398, y=w397) -> (x .and. y?=w395:bool)
        n458 = And(x=w400, y=w399) -> (x .and. y?=w396:bool)
        n459 = And(x=w395, y=w396) -> (x .and. y?=w376:bool)
        n460 = Add(x=w412, y=w413) -> (x+y=w411:T3)
        n461 = Add(x=w414, y=w349) -> (x+y=w371:T3)
        n462 = Less?(x=w413, y=w371) -> (x < y?=w409:cluster{bool, bool})
        n463 = Not(x=w376) -> (.not. x?=w378:bool)
        n464 = Greater?(x=w411, y=w349) -> (0:w410:cluster{bool, bool})
        n465 = Unbundle(w409) -> (w405:bool, w406:bool)
        n466 = Unbundle(w410) -> (w403:bool, w404:bool)
        n467 = property on="disco1" class="Bool (strict)"() -> ("Bounds"=w374:T3)  [unwired: 2 in, 2 out]
        n468 = property on="disco1" class="Bool (strict)"() -> ("Position"=w373:T1)  [unwired: 2 in, 2 out]
        n469 = Unbundle(w349) -> ("Left"=w366:i32)  [unwired: 1 out]
        n470 = And(x=w405, y=w406) -> (x .and. y?=w408:bool)
        n471 = And(x=w403, y=w404) -> (x .and. y?=w407:bool)
        n472 = Unbundle(w373) -> ("Left"=w365:i32)  [unwired: 1 out]
        n473 = Add(x=w374, y=w373) -> (x+y=w372:T3)
        n474 = Add(x=w365, y=30) -> (x+y=w363:i32)
        n475 = And(x=w408, y=w407) -> (x .and. y?=w375:bool)
        n476 = Unbundle(w372) -> ("Width"=w361:u32)  [unwired: 1 out]
        n477 = Greater?(x=w363, y=w366) -> (0:w369:bool)
        n478 = Subtract(x=w361, y=u32 30) -> (x-y=w362:u32)
        n479 = Not(x=w375) -> (.not. x?=w415:bool)
        n480 = Unbundle(w371) -> ("Width"=w370:u32)  [unwired: 1 out]
        n481 = Less?(x=w362, y=w370) -> (x < y?=w368:bool)
        n482 = And(x=w369, y=w368) -> (x .and. y?=w367:bool)
        n483 = Greater?(x=w350, y=w349) -> (0:w352:cluster{bool, bool})
        n484 = Unbundle(w352) -> (w354:bool, w355:bool)
        n485 = Less?(x=w350, y=w348) -> (x < y?=w353:cluster{bool, bool})
        n486 = And(x=w354, y=w355) -> (x .and. y?=w359:bool)
        n487 = Unbundle(w353) -> (w356:bool, w357:bool)
        n488 = Compound Arithmetic op=XOR(w416, w378, w415, w367) -> (w418:bool)
        n489 = And(x=w356, y=w357) -> (x .and. y?=w358:bool)
        n490 = And(x=w358, y=w359) -> (x .and. y?=w351:bool)
        n491 = case shown="False" w418 {
          tunnel: [FALSE ("Accepted?") TRUE ("Accepted?")] -> w417
          tunnel: w351 -> [w419 _]
          frame False {
            n492 = case shown="True" w419 {
              frame False {
              }
              frame True {
                n493 = local read "# de movimientos"() -> (w423:dbl)
                n494 = Wait (ms)(milliseconds to wait=u32 10) -> ()  [unwired: 1 out]
                n495 = Add(x=w423, y=1.0) -> (x+y=w424:dbl)
                n496 = local write "# de movimientos"(w424) -> ()
              }
            }
          }
          frame True {
            n497 = local read "Position 2"() -> (w426:T1)
            n498 = property on="disco2" class="Bool (strict)"("Position"=w426) -> ()  [unwired: 2 in, 2 out]
          }
        }
        n499 = Exclusive Or(1:w417, 2:w418) -> (0:w379:bool)
      }
      event Mouse Down {
        n500 = event-data() -> ("Coords"=w429:T2)  [unwired: 1 in, 7 out]
        n501 = property on="disco2" class="Bool (strict)"() -> ("Bounds"=w431:T3)  [unwired: 2 in, 2 out]
        n502 = property on="disco2" class="Bool (strict)"() -> ("Position"=w430:T1)  [unwired: 2 in, 2 out]
        "Position 2" <- w430
        n503 = property on="disco1" class="Bool (strict)"() -> ("Bounds"=w444:T3)  [unwired: 2 in, 2 out]
        n504 = property on="disco1" class="Bool (strict)"() -> ("Position"=w443:T1)  [unwired: 2 in, 2 out]
        n505 = Unbundle(w430) -> ("Left"=w441:i32, "Top"=w435:i32)
        n506 = Add(x=w430, y=w431) -> (x+y=w439:T3)
        n507 = Add(x=w443, y=w444) -> (x+y=w440:T3)
        n508 = Unbundle(w443) -> ("Left"=w442:i32, "Top"=w436:i32)
        n509 = Unbundle(w439) -> ("Width"=w437:u32)  [unwired: 1 out]
        n510 = Unbundle(w440) -> ("Width"=w438:u32)  [unwired: 1 out]
        n511 = Greater?(x=w442, y=w441) -> (0:w434:bool)
        n512 = Less?(x=w438, y=w437) -> (x < y?=w433:bool)
        n513 = Less?(x=w436, y=w435) -> (x < y?=w432:bool)
        n514 = Compound Arithmetic op=AND(w434, w433, w432) -> (w427:bool)
        n515 = case shown="False" w427 {
          tunnel: w429 -> [w446 _]
          tunnel: [w449 FALSE] -> w428
          tunnel: w431 -> [w448 _]
          tunnel: w430 -> [w447 _]
          tunnel: w429 -> [w445 _]
          frame False {
            n516 = Greater?(x=w445, y=w447) -> (0:w457:cluster{bool, bool})
            n517 = Unbundle(w457) -> (w453:bool, w452:bool)
            n518 = Add(x=w447, y=w448) -> (x+y=w458:T3)
            n519 = And(x=w453, y=w452) -> (x .and. y?=w450:bool)
            n520 = Less?(x=w446, y=w458) -> (x < y?=w456:cluster{bool, bool})
            n521 = Unbundle(w456) -> (w455:bool, w454:bool)
            n522 = And(x=w455, y=w454) -> (x .and. y?=w451:bool)
            n523 = And(x=w450, y=w451) -> (x .and. y?=w449:bool)
          }
          frame True {
          }
        }
      }
    }
    n524 = event shown="[2] \"Pane\": Mouse Up" {
      selector: _ -> [_ _ _ _]
      dyn-events: _ -> [_ _ _ _]
      timeout: _ -> [_ _ _ _]
      tunnel: w15 -> [w254 w255 _ _]
      tunnel: [w254 w255 w277 w329] -> w14
      event Timeout {
        n525 = event-data() -> ()  [unwired: 1 in, 3 out]
      }
      event Mouse Move {
        n526 = event-data() -> ("Coords"=w256:T2)  [unwired: 1 in, 4 out]
        n527 = case shown="True" w255 {
          tunnel: w256 -> [_ w260]
          frame False {
          }
          frame True {
            n528 = property on="disco1" class="Bool (strict)"() -> ("Bounds"=w258:T3)  [unwired: 2 in, 2 out]
            n529 = Divide(x=w258, y=T3 {"Width"=2, "Height"=2}) -> (x/y=w259:cluster{"Width":dbl, "Height":dbl})
            n530 = Subtract(x=w260, y=w259) -> (x-y=w257:cluster{dbl, dbl})
            n531 = property on="disco1" class="Bool (strict)"("Position"=w257) -> ()  [unwired: 2 in, 2 out]
          }
        }
      }
      event Mouse Up {
        n532 = event-data() -> ("Coords"=w264:T2)  [unwired: 1 in, 7 out]
        n533 = property on="medio" class="Bool (strict)"() -> ("Bounds"=w310:T3)  [unwired: 2 in, 2 out]
        n534 = property on="medio" class="Bool (strict)"() -> ("Position"=w309:T1)  [unwired: 2 in, 2 out]
        n535 = property on="disco1" class="Bool (strict)"() -> ("Position"=w265:T1)  [unwired: 2 in, 2 out]
        n536 = property on="disco1" class="Bool (strict)"() -> ("Bounds"=w283:T3)  [unwired: 2 in, 2 out]
        n537 = Add(x=w310, y=w309) -> (x+y=w308:T3)
        n538 = Add(x=w283, y=w265) -> (x+y=w263:T3)
        n539 = Less?(x=w309, y=w263) -> (x < y?=w312:cluster{bool, bool})
        n540 = Greater?(x=w308, y=w265) -> (0:w311:cluster{bool, bool})
        n541 = Unbundle(w312) -> (w316:bool, w315:bool)
        n542 = Unbundle(w311) -> (w318:bool, w317:bool)
        n543 = And(x=w316, y=w315) -> (x .and. y?=w313:bool)
        n544 = And(x=w318, y=w317) -> (x .and. y?=w314:bool)
        n545 = property on="final" class="Bool (strict)"() -> ("Position"=w296:T1)  [unwired: 2 in, 2 out]
        n546 = property on="final" class="Bool (strict)"() -> ("Bounds"=w297:T3)  [unwired: 2 in, 2 out]
        n547 = And(x=w313, y=w314) -> (x .and. y?=w276:bool)
        n548 = Not(x=w276) -> (.not. x?=w280:bool)
        n549 = Add(x=w297, y=w296) -> (x+y=w307:T3)
        n550 = Add(x=w283, y=w265) -> (x+y=w304:T3)
        n551 = Less?(x=w296, y=w304) -> (x < y?=w305:cluster{bool, bool})
        n552 = Greater?(x=w307, y=w265) -> (0:w306:cluster{bool, bool})
        n553 = Unbundle(w305) -> (w300:bool, w301:bool)
        n554 = Unbundle(w306) -> (w298:bool, w299:bool)
        n555 = property on="inicio" class="Bool (strict)"() -> ("Bounds"=w285:T3)  [unwired: 2 in, 2 out]
        n556 = property on="inicio" class="Bool (strict)"() -> ("Position"=w284:T1)  [unwired: 2 in, 2 out]
        n557 = And(x=w300, y=w301) -> (x .and. y?=w303:bool)
        n558 = And(x=w298, y=w299) -> (x .and. y?=w302:bool)
        n559 = And(x=w303, y=w302) -> (x .and. y?=w275:bool)
        n560 = Not(x=w275) -> (.not. x?=w281:bool)
        n561 = Add(x=w285, y=w284) -> (x+y=w286:T3)
        n562 = Add(x=w283, y=w265) -> (x+y=w289:T3)
        n563 = Less?(x=w284, y=w289) -> (x < y?=w288:cluster{bool, bool})
        n564 = Greater?(x=w286, y=w265) -> (0:w287:cluster{bool, bool})
        n565 = Unbundle(w288) -> (w293:bool, w292:bool)
        n566 = Unbundle(w287) -> (w295:bool, w294:bool)
        n567 = Greater?(x=w264, y=w265) -> (0:w273:cluster{bool, bool})
        n568 = And(x=w293, y=w292) -> (x .and. y?=w290:bool)
        n569 = And(x=w295, y=w294) -> (x .and. y?=w291:bool)
        n570 = Unbundle(w273) -> (w271:bool, w270:bool)
        n571 = And(x=w290, y=w291) -> (x .and. y?=w274:bool)
        n572 = Less?(x=w264, y=w263) -> (x < y?=w272:cluster{bool, bool})
        n573 = Not(x=w274) -> (.not. x?=w282:bool)
        n574 = And(x=w271, y=w270) -> (x .and. y?=w266:bool)
        n575 = Unbundle(w272) -> (w269:bool, w268:bool)
        n576 = And(x=w269, y=w268) -> (x .and. y?=w267:bool)
        n577 = And(x=w267, y=w266) -> (x .and. y?=w262:bool)
        n578 = Compound Arithmetic op=XOR(w280, w281, w282) -> (w279:bool)
        n579 = case shown="False" w279 {
          tunnel: [FALSE ("Accepted?") TRUE ("Accepted?")] -> w278
          tunnel: w262 -> [w319 _]
          frame False {
            n580 = case shown="True" w319 {
              frame False {
              }
              frame True {
                n581 = local read "# de movimientos"() -> (w323:dbl)
                n582 = Wait (ms)(milliseconds to wait=u32 10) -> ()  [unwired: 1 out]
                n583 = Add(x=w323, y=1.0) -> (x+y=w324:dbl)
                n584 = local write "# de movimientos"(w324) -> ()
              }
            }
          }
          frame True {
            n585 = local read "Position 1"() -> (w326:T1)
            n586 = property on="disco1" class="Bool (strict)"("Position"=w326) -> ()  [unwired: 2 in, 2 out]
          }
        }
        n587 = Exclusive Or(1:w278, 2:w279) -> (0:w277:bool)
      }
      event Mouse Down {
        n588 = event-data() -> ("Coords"=w338:T2)  [unwired: 1 in, 7 out]
        n589 = property on="disco1" class="Bool (strict)"() -> ("Position"=w327:T1)  [unwired: 2 in, 2 out]
        "Position 1" <- w327
        n590 = property on="disco1" class="Bool (strict)"() -> ("Bounds"=w328:T3)  [unwired: 2 in, 2 out]
        n591 = Greater?(x=w338, y=w327) -> (0:w337:cluster{bool, bool})
        n592 = Unbundle(w337) -> (w333:bool, w332:bool)
        n593 = Add(x=w327, y=w328) -> (x+y=w339:T3)
        n594 = And(x=w333, y=w332) -> (x .and. y?=w330:bool)
        n595 = Less?(x=w338, y=w339) -> (x < y?=w336:cluster{bool, bool})
        n596 = Unbundle(w336) -> (w335:bool, w334:bool)
        n597 = And(x=w335, y=w334) -> (x .and. y?=w331:bool)
        n598 = And(x=w330, y=w331) -> (x .and. y?=w329:bool)
      }
    }
    n599 = case shown="True" "?" {
      frame False {
      }
      frame True {
        w218 = FALSE ("result")
        n600 = property on="solucion de inicio a final 3" class="Str"("Visible"=FALSE) -> ()  [unwired: 2 in, 2 out]
        n601 = case shown="5" "seleccione  # de discos:" {
          frame 0, Default {
          }
          frame 5 {
            n602 = property on="disco3" class="Bool (strict)"("Visible"=TRUE) -> ()  [unwired: 2 in, 2 out]
            n603 = property on="disco4" class="Bool (strict)"("Visible"=TRUE) -> ()  [unwired: 2 in, 2 out]
            n604 = property on="disco2" class="Bool (strict)"("Visible"=TRUE) -> ()  [unwired: 2 in, 2 out]
            n605 = property on="disco1" class="Bool (strict)"("Visible"=TRUE) -> ()  [unwired: 2 in, 2 out]
            n606 = property on="disco5" class="Bool (strict)"("Visible"=TRUE) -> ()  [unwired: 2 in, 2 out]
            n607 = property on="disco4" class="Bool (strict)"("Position"=T1 {"Left"=285, "Top"=429}) -> ()  [unwired: 2 in, 2 out]
            n608 = property on="disco5" class="Bool (strict)"("Position"=T1 {"Left"=271, "Top"=451}) -> ()  [unwired: 2 in, 2 out]
            n609 = property on="disco3" class="Bool (strict)"("Position"=T1 {"Left"=297, "Top"=405}) -> ()  [unwired: 2 in, 2 out]
            n610 = property on="disco2" class="Bool (strict)"("Position"=T1 {"Left"=309, "Top"=381}) -> ()  [unwired: 2 in, 2 out]
            n611 = property on="disco1" class="Bool (strict)"("Position"=T1 {"Left"=321, "Top"=356}) -> ()  [unwired: 2 in, 2 out]
          }
          frame 4 {
            n612 = property on="disco3" class="Bool (strict)"("Visible"=TRUE) -> ()  [unwired: 2 in, 2 out]
            n613 = property on="disco4" class="Bool (strict)"("Visible"=TRUE) -> ()  [unwired: 2 in, 2 out]
            n614 = property on="disco2" class="Bool (strict)"("Visible"=TRUE) -> ()  [unwired: 2 in, 2 out]
            n615 = property on="disco1" class="Bool (strict)"("Visible"=TRUE) -> ()  [unwired: 2 in, 2 out]
            n616 = property on="disco5" class="Bool (strict)"("Visible"=FALSE) -> ()  [unwired: 2 in, 2 out]
            n617 = property on="disco4" class="Bool (strict)"("Position"=T1 {"Left"=285, "Top"=441}) -> ()  [unwired: 2 in, 2 out]
            n618 = property on="disco5" class="Bool (strict)"("Position"=T1 {"Left"=69, "Top"=489}) -> ()  [unwired: 2 in, 2 out]
            n619 = property on="disco3" class="Bool (strict)"("Position"=T1 {"Left"=297, "Top"=417}) -> ()  [unwired: 2 in, 2 out]
            n620 = property on="disco2" class="Bool (strict)"("Position"=T1 {"Left"=309, "Top"=393}) -> ()  [unwired: 2 in, 2 out]
            n621 = property on="disco1" class="Bool (strict)"("Position"=T1 {"Left"=321, "Top"=368}) -> ()  [unwired: 2 in, 2 out]
          }
          frame 3 {
            n622 = property on="disco3" class="Bool (strict)"("Visible"=TRUE) -> ()  [unwired: 2 in, 2 out]
            n623 = property on="disco4" class="Bool (strict)"("Visible"=FALSE) -> ()  [unwired: 2 in, 2 out]
            n624 = property on="disco2" class="Bool (strict)"("Visible"=TRUE) -> ()  [unwired: 2 in, 2 out]
            n625 = property on="disco1" class="Bool (strict)"("Visible"=TRUE) -> ()  [unwired: 2 in, 2 out]
            n626 = property on="disco5" class="Bool (strict)"("Visible"=FALSE) -> ()  [unwired: 2 in, 2 out]
            n627 = property on="disco4" class="Bool (strict)"("Position"=T1 {"Left"=93, "Top"=477}) -> ()  [unwired: 2 in, 2 out]
            n628 = property on="disco5" class="Bool (strict)"("Position"=T1 {"Left"=81, "Top"=501}) -> ()  [unwired: 2 in, 2 out]
            n629 = property on="disco3" class="Bool (strict)"("Position"=T1 {"Left"=297, "Top"=441}) -> ()  [unwired: 2 in, 2 out]
            n630 = property on="disco2" class="Bool (strict)"("Position"=T1 {"Left"=309, "Top"=417}) -> ()  [unwired: 2 in, 2 out]
            n631 = property on="disco1" class="Bool (strict)"("Position"=T1 {"Left"=321, "Top"=392}) -> ()  [unwired: 2 in, 2 out]
          }
        }
        n632 = property on="solucion de inicio a final 4" class="Str"("Visible"=FALSE) -> ()  [unwired: 2 in, 2 out]
        n633 = local write "# de movimientos"(0.0 ("movimientos")) -> ()
        n634 = property on="solucion de inicio a final 5" class="Str"("Visible"=FALSE) -> ()  [unwired: 2 in, 2 out]
        n635 = property class="Str"("Visible"=w218) -> ()  [unwired: 2 in, 2 out]
        n636 = local write "result"(w218) -> ()
      }
    }
    n637 = local write "result"(FALSE ("result")) -> ()
    n638 = local read "seleccione  # de discos:"() -> (w9:u16)
    n639 = case shown="5" w9 {
      frame 0, Default {
      }
      frame 5 {
        n640 = property on="final" class="Bool (strict)"() -> ("Bounds"=w106:T3)  [unwired: 2 in, 2 out]
        n641 = property on="final" class="Bool (strict)"() -> ("Position"=w107:T1)  [unwired: 2 in, 2 out]
        n642 = property on="disco1" class="Bool (strict)"() -> ("Position"=w109:T1)  [unwired: 2 in, 2 out]
        n643 = property on="disco1" class="Bool (strict)"() -> ("Bounds"=w103:T3)  [unwired: 2 in, 2 out]
        n644 = property on="final" class="Bool (strict)"() -> ("Bounds"=w87:T3)  [unwired: 2 in, 2 out]
        n645 = property on="final" class="Bool (strict)"() -> ("Position"=w86:T1)  [unwired: 2 in, 2 out]
        n646 = property on="disco2" class="Bool (strict)"() -> ("Position"=w84:T1)  [unwired: 2 in, 2 out]
        n647 = property on="disco2" class="Bool (strict)"() -> ("Bounds"=w90:T3)  [unwired: 2 in, 2 out]
        n648 = Add(x=w106, y=w107) -> (x+y=w108:T3)
        n649 = Add(x=w87, y=w86) -> (x+y=w85:T3)
        n650 = Add(x=w103, y=w109) -> (x+y=w110:T3)
        n651 = Add(x=w90, y=w84) -> (x+y=w83:T3)
        n652 = Less?(x=w107, y=w110) -> (x < y?=w104:cluster{bool, bool})
        n653 = Less?(x=w86, y=w83) -> (x < y?=w89:cluster{bool, bool})
        n654 = Greater?(x=w108, y=w109) -> (0:w105:cluster{bool, bool})
        n655 = Greater?(x=w85, y=w84) -> (0:w88:cluster{bool, bool})
        n656 = Unbundle(w104) -> (w100:bool, w99:bool)
        n657 = Unbundle(w105) -> (w98:bool, w97:bool)
        n658 = Unbundle(w89) -> (w93:bool, w94:bool)
        n659 = Unbundle(w88) -> (w95:bool, w96:bool)
        n660 = And(x=w100, y=w99) -> (x .and. y?=w102:bool)
        n661 = And(x=w98, y=w97) -> (x .and. y?=w101:bool)
        n662 = And(x=w93, y=w94) -> (x .and. y?=w91:bool)
        n663 = And(x=w95, y=w96) -> (x .and. y?=w92:bool)
        n664 = And(x=w102, y=w101) -> (x .and. y?=w68:bool)
        n665 = And(x=w91, y=w92) -> (x .and. y?=w67:bool)
        n666 = property on="final" class="Bool (strict)"() -> ("Bounds"=w78:T3)  [unwired: 2 in, 2 out]
        n667 = property on="final" class="Bool (strict)"() -> ("Position"=w79:T1)  [unwired: 2 in, 2 out]
        n668 = property on="disco3" class="Bool (strict)"() -> ("Position"=w81:T1)  [unwired: 2 in, 2 out]
        n669 = property on="disco3" class="Bool (strict)"() -> ("Bounds"=w75:T3)  [unwired: 2 in, 2 out]
        n670 = property on="final" class="Bool (strict)"() -> ("Bounds"=w56:T3)  [unwired: 2 in, 2 out]
        n671 = property on="final" class="Bool (strict)"() -> ("Position"=w55:T1)  [unwired: 2 in, 2 out]
        n672 = property on="disco4" class="Bool (strict)"() -> ("Position"=w53:T1)  [unwired: 2 in, 2 out]
        n673 = property on="disco4" class="Bool (strict)"() -> ("Bounds"=w59:T3)  [unwired: 2 in, 2 out]
        n674 = Add(x=w78, y=w79) -> (x+y=w80:T3)
        n675 = Add(x=w75, y=w81) -> (x+y=w82:T3)
        n676 = Add(x=w56, y=w55) -> (x+y=w54:T3)
        n677 = Add(x=w59, y=w53) -> (x+y=w52:T3)
        n678 = Less?(x=w79, y=w82) -> (x < y?=w76:cluster{bool, bool})
        n679 = Less?(x=w55, y=w52) -> (x < y?=w58:cluster{bool, bool})
        n680 = Greater?(x=w80, y=w81) -> (0:w77:cluster{bool, bool})
        n681 = Greater?(x=w54, y=w53) -> (0:w57:cluster{bool, bool})
        n682 = Unbundle(w76) -> (w72:bool, w71:bool)
        n683 = Unbundle(w77) -> (w70:bool, w69:bool)
        n684 = Unbundle(w58) -> (w62:bool, w63:bool)
        n685 = Unbundle(w57) -> (w64:bool, w65:bool)
        n686 = And(x=w72, y=w71) -> (x .and. y?=w74:bool)
        n687 = And(x=w70, y=w69) -> (x .and. y?=w73:bool)
        n688 = And(x=w62, y=w63) -> (x .and. y?=w60:bool)
        n689 = And(x=w64, y=w65) -> (x .and. y?=w61:bool)
        n690 = And(x=w74, y=w73) -> (x .and. y?=w66:bool)
        n691 = And(x=w60, y=w61) -> (x .and. y?=w37:bool)
        n692 = property on="final" class="Bool (strict)"() -> ("Bounds"=w47:T3)  [unwired: 2 in, 2 out]
        n693 = property on="final" class="Bool (strict)"() -> ("Position"=w48:T1)  [unwired: 2 in, 2 out]
        n694 = property on="disco5" class="Bool (strict)"() -> ("Position"=w50:T1)  [unwired: 2 in, 2 out]
        n695 = property on="disco5" class="Bool (strict)"() -> ("Bounds"=w44:T3)  [unwired: 2 in, 2 out]
        n696 = Add(x=w47, y=w48) -> (x+y=w49:T3)
        n697 = Add(x=w44, y=w50) -> (x+y=w51:T3)
        n698 = Less?(x=w48, y=w51) -> (x < y?=w45:cluster{bool, bool})
        n699 = Greater?(x=w49, y=w50) -> (0:w46:cluster{bool, bool})
        n700 = Unbundle(w45) -> (w41:bool, w40:bool)
        n701 = Unbundle(w46) -> (w39:bool, w38:bool)
        n702 = And(x=w41, y=w40) -> (x .and. y?=w43:bool)
        n703 = And(x=w39, y=w38) -> (x .and. y?=w42:bool)
        n704 = And(x=w43, y=w42) -> (x .and. y?=w36:bool)
        n705 = Compound Arithmetic op=AND(w68, w67, w66, w37, w36) -> (w35:bool)
        n706 = local write "result"(w35) -> ()
        n707 = property class="Str"("Visible"=w35) -> ()  [unwired: 2 in, 2 out]
      }
      frame 4 {
        n708 = property on="final" class="Bool (strict)"() -> ("Bounds"=w167:T3)  [unwired: 2 in, 2 out]
        n709 = property on="final" class="Bool (strict)"() -> ("Position"=w168:T1)  [unwired: 2 in, 2 out]
        n710 = property on="disco1" class="Bool (strict)"() -> ("Position"=w170:T1)  [unwired: 2 in, 2 out]
        n711 = property on="disco1" class="Bool (strict)"() -> ("Bounds"=w164:T3)  [unwired: 2 in, 2 out]
        n712 = property on="final" class="Bool (strict)"() -> ("Bounds"=w148:T3)  [unwired: 2 in, 2 out]
        n713 = property on="final" class="Bool (strict)"() -> ("Position"=w147:T1)  [unwired: 2 in, 2 out]
        n714 = property on="disco2" class="Bool (strict)"() -> ("Position"=w145:T1)  [unwired: 2 in, 2 out]
        n715 = property on="disco2" class="Bool (strict)"() -> ("Bounds"=w151:T3)  [unwired: 2 in, 2 out]
        n716 = Add(x=w167, y=w168) -> (x+y=w169:T3)
        n717 = Add(x=w148, y=w147) -> (x+y=w146:T3)
        n718 = Add(x=w164, y=w170) -> (x+y=w171:T3)
        n719 = Add(x=w151, y=w145) -> (x+y=w144:T3)
        n720 = Less?(x=w168, y=w171) -> (x < y?=w165:cluster{bool, bool})
        n721 = Less?(x=w147, y=w144) -> (x < y?=w150:cluster{bool, bool})
        n722 = Greater?(x=w169, y=w170) -> (0:w166:cluster{bool, bool})
        n723 = Greater?(x=w146, y=w145) -> (0:w149:cluster{bool, bool})
        n724 = Unbundle(w165) -> (w161:bool, w160:bool)
        n725 = Unbundle(w166) -> (w159:bool, w158:bool)
        n726 = Unbundle(w150) -> (w154:bool, w155:bool)
        n727 = Unbundle(w149) -> (w156:bool, w157:bool)
        n728 = And(x=w161, y=w160) -> (x .and. y?=w163:bool)
        n729 = And(x=w159, y=w158) -> (x .and. y?=w162:bool)
        n730 = And(x=w154, y=w155) -> (x .and. y?=w152:bool)
        n731 = And(x=w156, y=w157) -> (x .and. y?=w153:bool)
        n732 = And(x=w163, y=w162) -> (x .and. y?=w129:bool)
        n733 = And(x=w152, y=w153) -> (x .and. y?=w128:bool)
        n734 = property on="final" class="Bool (strict)"() -> ("Bounds"=w139:T3)  [unwired: 2 in, 2 out]
        n735 = property on="final" class="Bool (strict)"() -> ("Position"=w140:T1)  [unwired: 2 in, 2 out]
        n736 = property on="disco4" class="Bool (strict)"() -> ("Position"=w142:T1)  [unwired: 2 in, 2 out]
        n737 = property on="disco4" class="Bool (strict)"() -> ("Bounds"=w136:T3)  [unwired: 2 in, 2 out]
        n738 = Add(x=w139, y=w140) -> (x+y=w141:T3)
        n739 = Add(x=w136, y=w142) -> (x+y=w143:T3)
        n740 = Less?(x=w140, y=w143) -> (x < y?=w137:cluster{bool, bool})
        n741 = Greater?(x=w141, y=w142) -> (0:w138:cluster{bool, bool})
        n742 = property on="final" class="Bool (strict)"() -> ("Bounds"=w117:T3)  [unwired: 2 in, 2 out]
        n743 = property on="final" class="Bool (strict)"() -> ("Position"=w116:T1)  [unwired: 2 in, 2 out]
        n744 = property on="disco3" class="Bool (strict)"() -> ("Position"=w114:T1)  [unwired: 2 in, 2 out]
        n745 = property on="disco3" class="Bool (strict)"() -> ("Bounds"=w120:T3)  [unwired: 2 in, 2 out]
        n746 = Unbundle(w137) -> (w133:bool, w132:bool)
        n747 = Unbundle(w138) -> (w131:bool, w130:bool)
        n748 = And(x=w133, y=w132) -> (x .and. y?=w135:bool)
        n749 = And(x=w131, y=w130) -> (x .and. y?=w134:bool)
        n750 = Add(x=w117, y=w116) -> (x+y=w115:T3)
        n751 = Add(x=w120, y=w114) -> (x+y=w113:T3)
        n752 = And(x=w135, y=w134) -> (x .and. y?=w127:bool)
        n753 = Less?(x=w116, y=w113) -> (x < y?=w119:cluster{bool, bool})
        n754 = Greater?(x=w115, y=w114) -> (0:w118:cluster{bool, bool})
        n755 = Unbundle(w119) -> (w123:bool, w124:bool)
        n756 = Unbundle(w118) -> (w125:bool, w126:bool)
        n757 = And(x=w123, y=w124) -> (x .and. y?=w121:bool)
        n758 = And(x=w125, y=w126) -> (x .and. y?=w122:bool)
        n759 = And(x=w121, y=w122) -> (x .and. y?=w112:bool)
        n760 = Compound Arithmetic op=AND(w129, w128, w127, w112) -> (w111:bool)
        n761 = local write "result"(w111) -> ()
        n762 = property class="Str"("Visible"=w111) -> ()  [unwired: 2 in, 2 out]
      }
      frame 3 {
        n763 = property on="final" class="Bool (strict)"() -> ("Bounds"=w213:T3)  [unwired: 2 in, 2 out]
        n764 = property on="final" class="Bool (strict)"() -> ("Position"=w214:T1)  [unwired: 2 in, 2 out]
        n765 = property on="disco1" class="Bool (strict)"() -> ("Position"=w216:T1)  [unwired: 2 in, 2 out]
        n766 = property on="disco1" class="Bool (strict)"() -> ("Bounds"=w210:T3)  [unwired: 2 in, 2 out]
        n767 = property on="final" class="Bool (strict)"() -> ("Bounds"=w194:T3)  [unwired: 2 in, 2 out]
        n768 = property on="final" class="Bool (strict)"() -> ("Position"=w193:T1)  [unwired: 2 in, 2 out]
        n769 = property on="disco2" class="Bool (strict)"() -> ("Position"=w191:T1)  [unwired: 2 in, 2 out]
        n770 = property on="disco2" class="Bool (strict)"() -> ("Bounds"=w197:T3)  [unwired: 2 in, 2 out]
        n771 = Add(x=w213, y=w214) -> (x+y=w215:T3)
        n772 = Add(x=w194, y=w193) -> (x+y=w192:T3)
        n773 = Add(x=w210, y=w216) -> (x+y=w217:T3)
        n774 = Add(x=w197, y=w191) -> (x+y=w190:T3)
        n775 = Less?(x=w214, y=w217) -> (x < y?=w211:cluster{bool, bool})
        n776 = Less?(x=w193, y=w190) -> (x < y?=w196:cluster{bool, bool})
        n777 = Greater?(x=w215, y=w216) -> (0:w212:cluster{bool, bool})
        n778 = Greater?(x=w192, y=w191) -> (0:w195:cluster{bool, bool})
        n779 = Unbundle(w211) -> (w207:bool, w206:bool)
        n780 = Unbundle(w212) -> (w205:bool, w204:bool)
        n781 = Unbundle(w196) -> (w200:bool, w201:bool)
        n782 = Unbundle(w195) -> (w202:bool, w203:bool)
        n783 = And(x=w207, y=w206) -> (x .and. y?=w209:bool)
        n784 = And(x=w205, y=w204) -> (x .and. y?=w208:bool)
        n785 = And(x=w200, y=w201) -> (x .and. y?=w198:bool)
        n786 = And(x=w202, y=w203) -> (x .and. y?=w199:bool)
        n787 = And(x=w209, y=w208) -> (x .and. y?=w175:bool)
        n788 = And(x=w198, y=w199) -> (x .and. y?=w174:bool)
        n789 = property on="final" class="Bool (strict)"() -> ("Bounds"=w185:T3)  [unwired: 2 in, 2 out]
        n790 = property on="final" class="Bool (strict)"() -> ("Position"=w186:T1)  [unwired: 2 in, 2 out]
        n791 = property on="disco3" class="Bool (strict)"() -> ("Position"=w188:T1)  [unwired: 2 in, 2 out]
        n792 = property on="disco3" class="Bool (strict)"() -> ("Bounds"=w182:T3)  [unwired: 2 in, 2 out]
        n793 = Add(x=w185, y=w186) -> (x+y=w187:T3)
        n794 = Add(x=w182, y=w188) -> (x+y=w189:T3)
        n795 = Less?(x=w186, y=w189) -> (x < y?=w183:cluster{bool, bool})
        n796 = Greater?(x=w187, y=w188) -> (0:w184:cluster{bool, bool})
        n797 = Unbundle(w183) -> (w179:bool, w178:bool)
        n798 = Unbundle(w184) -> (w177:bool, w176:bool)
        n799 = And(x=w179, y=w178) -> (x .and. y?=w181:bool)
        n800 = And(x=w177, y=w176) -> (x .and. y?=w180:bool)
        n801 = And(x=w181, y=w180) -> (x .and. y?=w173:bool)
        n802 = Compound Arithmetic op=AND(w175, w174, w173) -> (w172:bool)
        "result" <- w172
        n803 = property class="Str"("Visible"=w172) -> ()  [unwired: 2 in, 2 out]
      }
    }
    n804 = Wait (ms)(milliseconds to wait=u32 10) -> ()  [unwired: 1 out]
    n805 = Wait (ms)(milliseconds to wait=u32 10) -> ()  [unwired: 1 out]
    n806 = case shown="True" "?" {
      frame False {
      }
      frame True {
        n807 = local read "seleccione  # de discos:"() -> (w25:u16)
        n808 = case shown="5" w25 {
          frame 0, Default {
          }
          frame 5 {
            n809 = property on="solucion de inicio a final 5" class="Str"("Visible"=TRUE) -> ()  [unwired: 2 in, 2 out]
            n810 = property on="solucion de inicio a final 3" class="Str"("Visible"=FALSE) -> ()  [unwired: 2 in, 2 out]
            n811 = property on="solucion de inicio a final 4" class="Str"("Visible"=FALSE) -> ()  [unwired: 2 in, 2 out]
          }
          frame 4 {
            n812 = property on="solucion de inicio a final 5" class="Str"("Visible"=FALSE) -> ()  [unwired: 2 in, 2 out]
            n813 = property on="solucion de inicio a final 3" class="Str"("Visible"=FALSE) -> ()  [unwired: 2 in, 2 out]
            n814 = property on="solucion de inicio a final 4" class="Str"("Visible"=TRUE) -> ()  [unwired: 2 in, 2 out]
          }
          frame 3 {
            n815 = property on="solucion de inicio a final 5" class="Str"("Visible"=FALSE) -> ()  [unwired: 2 in, 2 out]
            n816 = property on="solucion de inicio a final 3" class="Str"("Visible"=TRUE) -> ()  [unwired: 2 in, 2 out]
            n817 = property on="solucion de inicio a final 4" class="Str"("Visible"=FALSE) -> ()  [unwired: 2 in, 2 out]
          }
        }
      }
    }
  }
  n818 = property class="Str"("Visible"=FALSE ("result")) -> ()  [unwired: 2 in, 2 out]
  "# de movimientos" <- 0.0 ("movimientos")
  "solucion de inicio a final 3" <- "-disco uno a final\n-disco dos a medio\n-disco uno a medio\n-disco tres a final\n-disco uno a inicio\n-disco dos a final\ndisco uno a final" ("solucion de inicio a final 3")
  "solucion de inicio a final 5" <- "-disco uno a final\n-disco dos a medio\n-disco uno a medio\n-disco tres a final\n-disco uno a inicio\n-disco dos a final\n-disco uno a final\n-disco cuatro a medio\n-disco uno a medio\n-disco dos a inicio\n-disco uno a inicio\n-disco tres a medio\n-disco uno a final\n-disco dos a medio\n-disco uno a medio\n-disco cinco a final\n-disco uno a inicio\n-disco dos a final\n-disco uno a final\n-disco tres a inicio\n-disco uno a medio\n-disco dos a inicio\n-disco uno a inicio\n-disco cuatro a final\n-disco uno a final\n-disco dos a medio\n-disco uno a medio\n-disco tres a final\n-disco uno a inicio\n-disco dos a final\n-disco uno a final" ("solucion de inicio a final 5")
  "solucion de inicio a final 4" <- "-disco uno a medio\n-disco medio a final\n-disco uno a final\n-disco tres a medio\n-disco uno a inicio\n-disco dos a medio\n-disco uno a medio\n-disco cuatro a final\n-disco uno a final\n-disco dos a inicio\n-disco uno a inicio\n-disco tres a final\n-disco uno medio\n-disco dos a final\n-disco uno a final\n" ("solucion de inicio a final 4")
